vi "new_main_save_encoder.vi"() -> ()   [LabVIEW 2019]
uses:
  <vilib>/vision/Image Controls.llb/IMAQ Image.ctl
  <vilib>/Utility/error.llb/DialogType.ctl
  <vilib>/DAQmx/write.llb/DAQmx Write (Digital Bool 1Line 1Point).vi
  <vilib>/DAQmx/write.llb/DAQmx Write (Counter Frequency 1Chan 1Samp).vi
  <vilib>/Analysis/baseanly.llb/Mean (DBL).vi
  <vilib>/DAQmx/miscellaneous.llb/DAQmx Fill In Error Info.vi
  <vilib>/Utility/file.llb/Write Delimited Spreadsheet (DBL).vi
  <vilib>/addons/control/pid/pid.llb/PID (DBL).vi
  <vilib>/addons/control/pid/pid.llb/PID Gain Schedule (DBL).vi
  <vilib>/DAQmx/create/channels.llb/DAQmx Create Channel (CO-Pulse Generation-Frequency).vi
  <vilib>/DAQmx/configure/timing.llb/DAQmx Timing (Implicit).vi
  <vilib>/vision/driver/NI_Vision_Acquisition_Software.lvlib
  <vilib>/userDefined/High Color/IMAQdx.ctl
  <instrlib>/Yokogawa PZ4000/Yokogawa PZ4000.lvlib
  <vilib>/Analysis/NI_AALBase.lvlib
  <vilib>/addons/control/pid/NI_PID_pid.lvlib
  <instrlib>/Agilent 34970/Agilent 34970.lvlib
  <instrlib>/Yokogawa WT200 Series/Yokogawa WT200 Series.lvlib
  <resource>/objmgr/daqmx.rc
panel:
  in  "encoder files":u32=10
  in  "Salvar encoder":bool
  in  "encoder wait":u32=200
  out "T end ensaio":dbl format="%_19f"
  out "T init ensaio":dbl format="%_19f"
  out "save name":string
  out "Error Out":T1
  out "Torque à vazio":dbl format="%_19f"
  out "error out 3":errorcluster
  out "temperature array cluster":T2
  out "temperature num cluster":T3
  out "watt num cluster":T4
  out "var controle rpm":u16
  out "var controle torque":dbl format="%.2f"
  out "error out 2":errorcluster
  out "watt array cluster":T5
  out "rpm array cluster":T6
  out "rpm values cluster":T7
  out "stop aquisition?":bool
  out "torque values cluster":T8
  out "torque array cluster":T9
  out "lim sup rpm":dbl=250000.0 format="%#_13g"
  out "lim inf rpm":dbl=250000.0 format="%#_13g"
  out "lim inf torque":dbl=250000.0 format="%#_13g"
  out "lim sup torque":dbl=250000.0 format="%#_13g"
  out "t0 ensaio":dbl format="%_19f"
  out "error out":errorcluster
  out "Referência entrada (RPM)":dbl
  out "RPM":dbl
  out "Image Out":T10
  out "torque mean":dbl format="%0.2f"
  out "semaforo medição":T11
  out "Status de execução":string
  out "eixo girando?":bool
  out "Referência entrada (mN.m)":dbl
  out "ME":enum16{"Stand-by", "Ensaiando", "Saindo"}(ring)
  in  "stop geral":bool
  in  "Tab Control":T12(tab)
  in  "manter na condição após ensaio?":bool
  in  "T aquisição":dbl=10.0 format="%#_13g"
  in  "name or relative path":string
  out "Power XY":cluster{dbl[], dbl[]}(graph)
  out "Torque XY":cluster{"t":dbl[], dbl[]}[](graph)
  in  "Torque (mN.m)":dbl min=0.0 max=500.0 step=0.1
  in  "Velocidade angular (RPM)":dbl=1000.0 min=1000.0 max=3600.0 step=0.1
  out "Descrição":string
  in  "Lista de ensaios":T13(ring)
  in  "Iniciar ensaio":bool
  in  "stop ensaio":bool
  in  "Ensaiando?":bool
  out "RPM XY":cluster{"t":dbl[], dbl[]}[](graph)
  in  "Salvar dados":bool
  in  "Tab Control 5":enum32{"RPM", "Torque", "Temperatura"}(tab)
  out "encoder saved":i32
  out "Waveform RPM":dynamicdata(graph)
  out "Waveform Torque":dynamicdata(graph)
  out "Chart Temperatura":cluster{dbl, dbl, dbl, dbl, dbl, dbl}(graph)
  in  "Tab Control 4":enum32{"Numeric - WT230", "Waveform - PZ4000"}(tab)
  out "Chart potencia numeric":T14(graph)
  out "Chart corrente numeric":cluster{"I(A)":dbl, "I(B)":dbl, "I(E)":dbl}(graph)
  out "Chart tensão numeric":cluster{"V(A)":dbl, "V(B)":dbl, "V(E)":dbl}(graph)
  out "Chart Potencia":cluster{dbl, dbl, dbl, dbl}(graph)
  out "Corrente":dbl[][](graph)
  out "Tensão":dbl[][](graph)
  in  "Tab Control 3":T15(tab)
  in  "Tab Control 6":T16(tab)
  in  "Parar motor":bool
  in  "Enviar velocidade":bool
  in  "Velocidade (RPM)":u16=1000 min=1000 max=10000 step=100
  in  "Frequência PWM":u16(ring) items=["2000 Hz", "3600 Hz", "5000 Hz", "8000 Hz"]
  in  "Enviar frequência":bool
  in  "Modo PWM":u16(ring) items=["Standard", "Complete", "Symmetric", "Anti Symmetric"]
  in  "Enviar modo":bool
  out "Tradução":string
  in  "Envia mensagem":bool
  in  "Mensagem":T17(ring)=enum."Read power"
  out "Resposta":string
  in  "Seta carga":bool
  in  "Liga saída":bool
  out "Corrente de saída":dbl format="%.4f"
  out "Tensão de saída":dbl format="%.4f"
  in  "Limite de tensão":dbl=15.0 min=0.0 max=17.0 step=0.5 format="%.4f"
  in  "Limite de corrente":dbl=0.3000000000000001 min=0.0 max=0.4 step=0.01 format="%.4f"
  in  "Tempo de aquisição":u16(ring)=12 items=["1ksec", "400sec", "200sec", "100sec", "40sec", "20sec", "10sec", "4sec", "2sec", "1sec", "400msec", "200msec", "100msec", "40msec", "20msec", "10msec", "4msec", "2msec", "1msec", "400usec", "200usec", "100usec", "40usec", "20usec", "10usec"]
  in  "Waveform?":bool
  in  "Filtro de linha":u16(ring) items=["OFF", "500Hz", "20kHz", "1MHz"]
  in  "Média":u16(ring)=6 items=["2", "4", "8", "16", "32", "64", "OFF"]
  in  "dt integracao":dbl=1.0 format="%#_13g"
  in  "Realiza medição PZ4000":bool
  in  "Medição contínua? PZ4000":bool
  in  "Realiza medição WT230":bool
  in  "Medição contínua? WT230":bool
  in  "Tempo de integração (s)":u32=10 min=1 max=60 step=1
  in  "Liga aquecedor":bool
  in  "Frequency":dbl=1.0 format="%.6f"
  in  "Duty Cycle":dbl=0.225 format="%.6f"
  out "Chart RPM":T18(graph)
  in  "stop manual":bool
  out "Chart Torque":T19(graph)
  in  "Tab Control 2":enum32{"Torque", "Velocidade", "Torque GS"}(tab)
  in  "Habilitar (Torque)":bool
  in  "Referência (mN.m)":dbl min=0.0 max=500.0 step=0.1
  in  "Setar referência (Torque)":bool
  in  "PID Torque":T20={"proportional gain (Kc)"=0.0002, "integral time (Ti, min)"=0.005, "derivative time (Td, min)"=0.0}
  out "torque em rp?":bool
  in  "PID RPM":T20={"proportional gain (Kc)"=0.05, "integral time (Ti, min)"=0.005, "derivative time (Td, min)"=0.0}
  in  "Referência (RPM)":dbl=1000.0 min=900.0 max=5000.0 step=0.1
  in  "Habilitar (RPM)":bool
  in  "Setar referência (RPM)":bool
  out "rpm em rp?":bool
  in  "PID gain schedule":T21(array[cluster])=[{"PID gains"={"proportional gain (Kc)"=0.000167, "integral time (Ti, min)"=0.0048, "derivative time (Td, min)"=0.0}, "max value"=75.0}] {"max value" format="%.2f"; "PID gains"."derivative time (Td, min)" format="%.7f"; "PID gains"."integral time (Ti, min)" format="%.7f"; "PID gains"."proportional gain (Kc)" format="%.7f"}
  in  "waveform file name":string="data_%d%m@%H%M%S.txt"
  in  "Salvar waveform":bool
  in  "Limpa gráficos":bool
  in  "Janela de dados (s)":dbl=600.0
  in  "Iluminação":bool
  out "Image":T10(plugin-control)
  in  "Margem RPM (%)":dbl=0.5 min=0.0 max=2.1 step=0.1
  in  "Margem torque (%)":dbl=0.4999999999999998 min=0.0 max=2.1 step=0.1
  in  "Parâmetros serial":T22={"Serial VCC"="COM5", "timeout"=2, "baud rate"=600, "flow control"=0, "data bits"=8, "parity"=enum."None", "stop bits"=10, "termination char"=FALSE} {"stop bits" items=["1.0"=10, "1.5"=15, "2.0"=20]; "flow control" items=["None", "XON/XOFF", "RTS/CTS", "XON/XOFF & RTS/CTS", "DTR/DSR", "XON/XOFF & DTR/DSR"]}
  in  "RPM Samples (n)":i32=25000
  in  "RPM Rate (Hz)":dbl=500000.0 format="%#_13g"
  in  "Torque Samples (n)":i32=25000
  in  "Torque Rate (Hz)":dbl=500000.0 format="%#_13g"
  in  "Array frequências":u16[](array[ring])=[0, 1, 2, 3] items=["2000 Hz", "3600 Hz", "5000 Hz", "8000 Hz"]
  in  "Array modos":u16[](array[ring])=[0, 2, 3] items=["Standard", "Complete", "Symmetric", "Anti Symmetric"]
  in  "format":string="%.10f"
  # "Parâmetros"
  # "Execução"
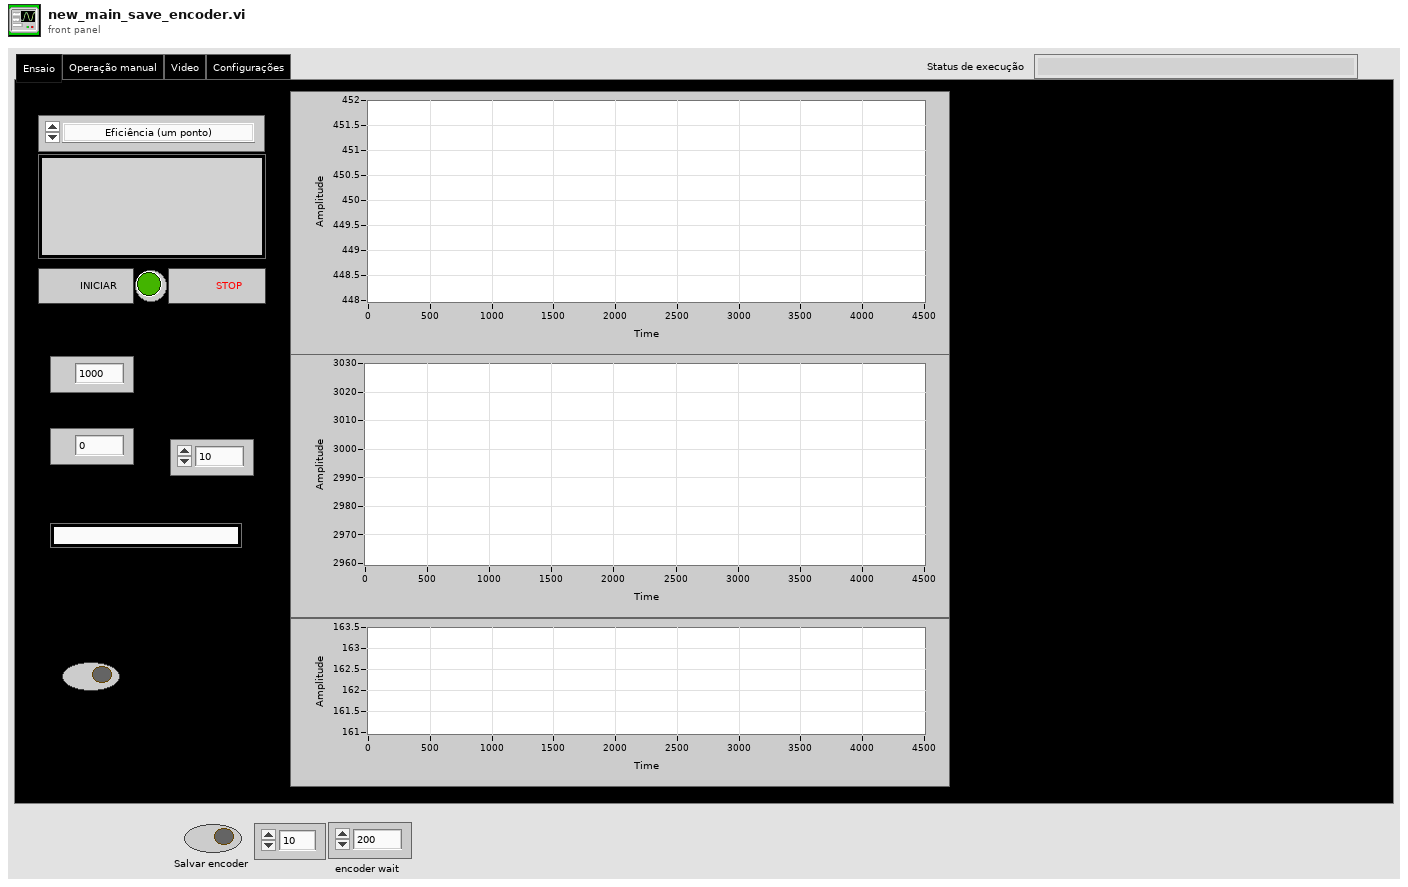
[diagram p1: front panel]
types:
  T1 = cluster{"status":bool, "code":i32, "message":string}
  T2 = cluster{"t":dbl[], "t1 bobina":dbl[], "t2 bobina":dbl[], "t freio":dbl[], "t rola frente":dbl[], "t rola tras":dbl[], "t amb":dbl[], "duty cycle":dbl[]}
  T3 = cluster{"t1 bobina":dbl, "t2 bobina":dbl, "t freio":dbl, "tempo":dbl, "t rola frente":dbl, "t rola tras":dbl, "t amb":dbl, "duty cycle":dbl}
  T4 = cluster{"V(A)":dbl, "I(A)":dbl, "V(B)":dbl, "I(B)":dbl, "PC(A)":dbl, "PC(B)":dbl, "PC(T)":dbl, "PL(T)":dbl, "PL(B)":dbl, "PL(A)":dbl, "V(E)":dbl, "PL(E)":dbl, "PC(E)":dbl, "I(E)":dbl, "t":dbl}
  T5 = cluster{"t":dbl[], "V(A)":dbl[], "I(A)":dbl[], "V(B)":dbl[], "I(B)":dbl[], "PC(A)":dbl[], "PC(B)":dbl[], "PC(T)":dbl[], "PL(T)":dbl[], "PL(B)":dbl[], "PL(A)":dbl[], "V(E)":dbl[], "PL(E)":dbl[], "PC(E)":dbl[], "I(E)":dbl[]}
  T6 = cluster{"t":dbl[], "rpm":dbl[], "ref":dbl[], "lim sup":dbl[], "lim inf":dbl[], "var contr":dbl[]}
  T7 = cluster{"relative seconds":dbl, "RPM":dbl, "Referência entrada (RPM)":dbl, "lim sup rpm":dbl, "lim inf rpm":dbl, "var controle rpm":dbl}
  T8 = cluster{"relative seconds":dbl, "mean":dbl, "Referência entrada (mN.m)":dbl, "lim sup torque":dbl, "lim inf torque":dbl, "var controle torque":dbl}
  T9 = cluster{"t":dbl[], "torque":dbl[], "ref":dbl[], "lim sup":dbl[], "lim inf":dbl[], "var contr":dbl[]}
  T10 = typedef "IMAQ Image.ctl" = refnum<image>
  T11 = typedef "Semaphore RefNum" = refnum<k1>
  T12 = enum32{"Ensaio", "Operação manual", "Video", "Configurações"}
  T13 = enum16{"Eficiência (um ponto)", "Eficiência (um ponto) v2", "Eficiência (múltiplos pontos)"}
  T14 = cluster{"PC(A)":dbl, "PC(B)":dbl, "PC(T)":dbl, "PL(A)":dbl, "PL(B)":dbl, "PL(T)":dbl, "PC(E)":dbl, "PL(E)":dbl}
  T15 = enum32{"Inversor", "Freio", "PZ4000", "WT230", "Aquecimento"}
  T16 = enum32{"Velocidade", "Frequência PWM", "Modo PWM"}
  T17 = enum16{"Read set speed", "Read operation status", "Read power", "Read starting trials", "Read bus voltage", "Read temperature", "Read power limitation", "Read PWM mode", "Read PWM frequency", "Read real speed"}
  T18 = cluster{"RPM":dbl, "Referência entrada (RPM)":dbl, "lim sup rpm":dbl, "lim inf rpm":dbl}
  T19 = cluster{"mean":dbl, "Referência entrada (mN.m)":dbl, "lim sup torque":dbl, "lim inf torque":dbl}
  T20 = cluster{"proportional gain (Kc)":dbl, "integral time (Ti, min)":dbl, "derivative time (Td, min)":dbl}
  T21 = cluster{"PID gains":cluster{"proportional gain (Kc)":dbl, "integral time (Ti, min)":dbl, "derivative time (Td, min)":dbl}, "max value":dbl}[]
  T22 = cluster{"Serial VCC":refnum<visa-resource-name>, "timeout":u32, "baud rate":u32, "flow control":u16, "data bits":u16, "parity":enum16{"None", "Odd", "Even", "Mark", "Space"}, "stop bits":u16, "termination char":bool}
  T23 = enum8{"Enabled", "Disabled", "Disabled and Grayed Out"}
  T24 = enum32{"Page Enabled", "Page Disabled", "Page Disabled & Grayed"}
  T25 = typedef "IMAQdx.ctl" = refnum<k21>
  T26 = enum16{"Start Comm.", "End Comm.", "Wait", "Send Static Message", "Set Speed"}
  T27 = enum16{"Thermocouple", "Thermistor", "RTD", "4-Wire RTD", "Default (Last)"}
  T28 = enum16{"Start Comm.", "End Comm.", "Wait", "Send Static Message", "Set Speed", "Set PWM Mode", "Set PWM Frequency"}
  T29 = enum16{"Read set speed", "Read operation status", "Read power", "Read starting trials", "Read bus voltage", "Read temperature", "Read power limitation", "Read PWM mode", "Read PWM frequency"}
  T30 = cluster{"mean":dbl, "Referência entrada (mN.m)":dbl, "lim sup torque":dbl, "lim inf torque":dbl}[]
  T31 = cluster{"relative seconds":dbl, dbl, "Referência entrada (mN.m)":dbl, "lim sup torque":dbl, "lim inf torque":dbl, "var controle torque":dbl}
  T32 = cluster{dbl, "Referência entrada (mN.m)":dbl, "lim sup torque":dbl, "lim inf torque":dbl}
  T33 = typedef "DialogType.ctl" = u16
  T34 = cluster{"relative seconds":dbl, "RPM":dbl, "Referência entrada (RPM)":dbl, "lim sup rpm":dbl, "lim inf rpm":dbl, "var controle rpm":u16}
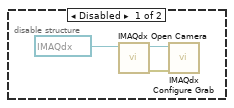
[diagram p3: hidden frame]
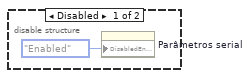
[diagram p4: hidden frame]
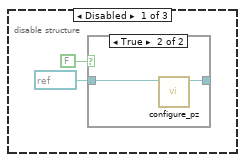
[diagram p5: hidden frame]
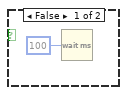
[diagram p8: hidden frame]
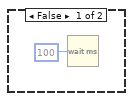
[diagram p9: hidden frame]
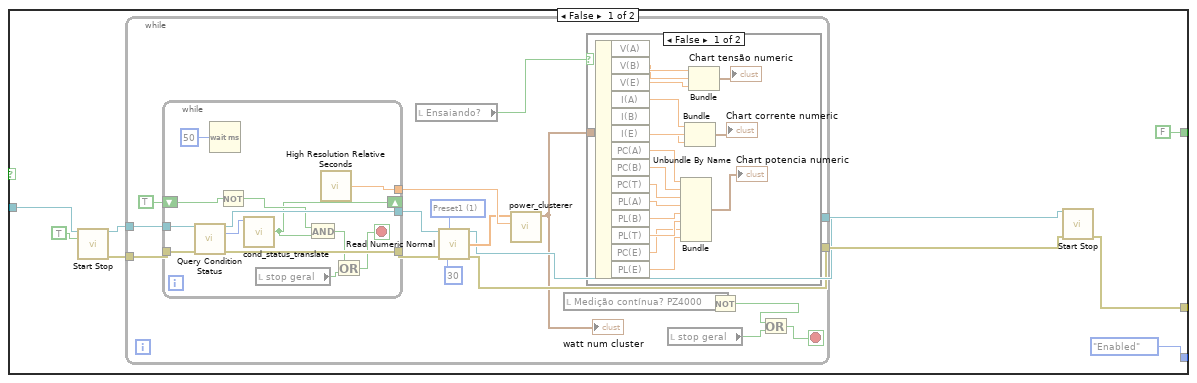
[diagram p10: hidden frame]
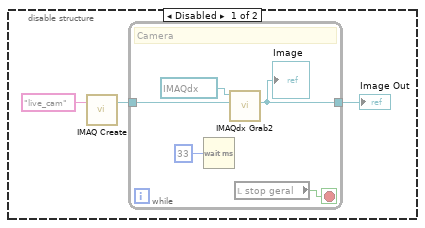
[diagram p13: hidden frame]
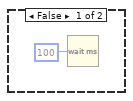
[diagram p14: hidden frame]
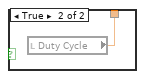
[diagram p16: hidden frame]
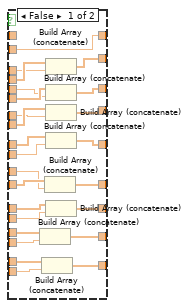
[diagram p18: hidden frame]
diagram:
  n1 = flat-sequence {
    frame #0 {
      "Status de execução" <- "Configurando" ("Status de execução")
      "ME" <- enum16{"Stand-by", "Ensaiando", "Saindo"}."Stand-by" ("ME")
      "Referência entrada (mN.m)" <- 0.0 ("Referência entrada")
      "Referência entrada (RPM)" <- 0.0 ("Referência entrada")
      "Torque à vazio" <- 0.0 ("Torque à vazio")
    }
    frame #1 {
      w11 = T8 {"relative seconds"=nan, "mean"=nan, "Referência entrada (mN.m)"=nan, "lim sup torque"=nan, "lim inf torque"=nan, "var controle torque"=nan} ("torque values cluster")
      w16 = T30 [] ("History Data")
      w21 = T23."Enabled" ("Disabled")
      w22 = 0.0 ("Referência")
      w27 = refnum<k21> "resfriamento_freio"  # DAQmx Task Name
      w6 = FALSE ("data")
      n2 = disable-structure shown="Disabled" {
        frame Disabled {
          n3 = case shown="True" FALSE ("configure?") {
            tunnel: [w52 w54] -> _
            tunnel: refnum<visa-resource-name> "PZ" ("VISA Refnum in") -> [w52 w53]
            frame False {
            }
            frame True {
              n4 = call "configure_pz.vi"("VISA Refnum in"=w53) -> ("VISA Refnum out"=w54:refnum<visa-resource-name>)  [unwired: 10 in]
            }
          }
        }
        frame Enabled {
        }
        frame Disabled {
          w58 = u16 9 items=["AUTO", "0.1", "0.2", "0.4", "1", "2", "4", "10", "20", "40", "100"] ("A Range (7:10)")
          w59 = u16 1 items=["5A", "20A", "Sensor"] ("A Terminal (0: 5A)")
          w60 = u16 6 items=["AUTO", "30", "60", "120", "200", "300", "600", "1200", "2000"] ("V Range (8: 2000)")
          n5 = call <instrlib>:"Initialize.vi"("VISA resource name"=refnum<visa-resource-name> "PZ" ("VISA Refnum in"), "Reset (T: Reset)"=FALSE) -> ("VISA resource name out"=w56:refnum<visa-resource-name>)  [unwired: 12 in, 1 out]
          n6 = call <instrlib>:"Config Voltage.vi"("VISA resource name"=w56, "V Range (8: 2000)"=w60) -> ("VISA resource name out"=w61:refnum<visa-resource-name>)  [unwired: 12 in, 1 out]
          n7 = call <instrlib>:"Config Current.vi"("VISA resource name"=w61, "A Terminal (0: 5A)"=w59, "A Range (7:10)"=w58) -> ()  [unwired: 11 in, 2 out]
        }
      }
      n8 = disable-structure shown="Disabled" {
        frame Disabled {
          w35 = refnum<k21> "iluminacao"  # DAQmx Task Name
          n9 = call <vilib>:"DAQmx Start Task.vi"("task/channels in"=w35) -> ("task out"=w36:refnum<k21>)  [unwired: 13 in, 1 out]
          n10 = call-poly <vilib>:"DAQmx Write.vi"("task/channels in"=w36, "data"=FALSE) -> ()  [unwired: 11 in, 3 out]
        }
        frame Enabled {
        }
      }
      n11 = local write "Referência (mN.m)"(w22) -> ()
      n12 = property on="Tab Control" class="TabCtl (strict)"() -> ("Pages"=w31:refnum<vi>[])  [unwired: 2 in, 2 out]
      n13 = local write "Referência (RPM)"(w22) -> ()
      n14 = Index Array(array=w31, index=1) -> (element=w32:refnum<vi>)
      n15 = property on="Chart Torque" class="WFChart (strict)"("History Data"=w16) -> ()  [unwired: 2 in, 2 out]
      n16 = property class="Page"(reference=w32, "PageEnb"=T24."Page Enabled" ("Page Enabled State")) -> ()  [unwired: 1 in, 2 out]
      n17 = property on="Chart RPM" class="WFChart (strict)"("History Data"=w16) -> ()  [unwired: 2 in, 2 out]
      n18 = local write "torque values cluster"(w11) -> ()
      n19 = local write "rpm values cluster"(w11) -> ()
      n20 = local write "watt num cluster"(T4 {"V(A)"=0.0, "I(A)"=0.0, "V(B)"=0.0, "I(B)"=0.0, "PC(A)"=0.0, "PC(B)"=0.0, "PC(T)"=0.0, "PL(T)"=0.0, "PL(B)"=0.0, "PL(A)"=0.0, "V(E)"=0.0, "PL(E)"=0.0, "PC(E)"=0.0, "I(E)"=0.0, "t"=0.0} ("watt num cluster")) -> ()
      n21 = disable-structure shown="Enabled" {
        frame Disabled {
          n22 = call <vilib>:"IMAQdx Open Camera.vi"("Session In"=T25 "cam0") -> ("error out"=w37:errorcluster, "Session Out"=w38:T25)  [unwired: 9 in]
          n23 = call <vilib>:"IMAQdx Configure Grab.vi"("error in"=w37, "Session In"=w38) -> ()  [unwired: 8 in, 2 out]
        }
        frame Enabled {
        }
      }
      n24 = flat-sequence {
        frame #0 {
          w41 = refnum<k21> "alimentacao_inversor"  # DAQmx Task Name
          n25 = call <vilib>:"DAQmx Start Task.vi"("task/channels in"=w41) -> ("task out"=w43:refnum<k21>)  [unwired: 13 in, 1 out]
          n26 = call-poly <vilib>:"DAQmx Write.vi"("task/channels in"=w43, "data"=TRUE) -> ()  [unwired: 11 in, 3 out]
        }
        frame #1 {
          n27 = Wait (ms)(milliseconds to wait=u32 3000) -> ()  [unwired: 1 out]
        }
        frame #2 {
          n28 = call "Serial_control.vi"("Função"=T26."Start Comm.", "comm cluster"="Parâmetros serial") -> ()  [unwired: 3 in, 4 out]
        }
        frame #3 {
          n29 = local read "Parâmetros serial"() -> (w48:T22)
          n30 = call "Serial_control.vi"("Enviar número"=u16 0, "Função"=T26."Set Speed", "comm cluster"=w48) -> ()  [unwired: 2 in, 4 out]
        }
      }
      n31 = call <vilib>:"Obtain Semaphore Reference.vi"() -> ("semaphore"=→"semaforo medição":T11)  [unwired: 5 in, 2 out]
      n32 = property on="Chart Potencia" class="WFChart (strict)"("History Data"=cluster{dbl, dbl, dbl, dbl}[] []) -> ()  [unwired: 2 in, 2 out]
      n33 = property on="Iniciar ensaio" class="Bool (strict)"("DisabledEnum"=T23."Enabled" ("Disabled")) -> ()  [unwired: 2 in, 2 out]
      n34 = disable-structure shown="Enabled" {
        frame Disabled {
          n35 = property on="Parâmetros serial" class="Clust (strict)"("DisabledEnum"=T23."Enabled" ("Disabled")) -> ()  [unwired: 2 in, 2 out]
        }
        frame Enabled {
        }
      }
      n36 = call <instrlib>:"GENie Initialize.vi"("Reset (T)"=TRUE, "VISA name"=refnum<visa-resource-name> "Lambda") -> ("error out"=w15:errorcluster, "VISA out"=w14:refnum<visa-resource-name>)  [unwired: 8 in]
      n37 = call <instrlib>:"Initialize.vi"("VISA Resource Name"=refnum<visa-resource-name> "Agilent" ("VISA AGILENT"), "Reset (T: Reset)"=TRUE) -> ()  [unwired: 12 in, 2 out]
      n38 = property on="Parâmetros serial" class="Clust (strict)"("DisabledEnum"=T23."Enabled" ("Disabled")) -> ()  [unwired: 2 in, 2 out]
      n39 = call <vilib>:"DAQmx Start Task.vi"("task/channels in"=w27) -> ("task out"=w26:refnum<k21>)  [unwired: 13 in, 1 out]
      n40 = call <instrlib>:"GENie Config Power-On State.vi"("error"=w15, "Power-On"=enum16{"Safe-Start", "Auto-Start"}."Safe-Start", "VISA"=w14) -> ()  [unwired: 7 in, 2 out]
      n41 = call-poly <vilib>:"DAQmx Write.vi"("task/channels in"=w26, "data"=FALSE) -> ()  [unwired: 11 in, 3 out]
      n42 = local write "Realiza medição PZ4000"(w6) -> ()
      n43 = local write "Realiza medição WT230"(w6) -> ()
      n44 = local write "Enviar velocidade"(w6) -> ()
      n45 = local write "stop manual"(w6) -> ()
      n46 = local write "stop ensaio"(w6) -> ()
      n47 = local write "Envia mensagem"(w6) -> ()
      n48 = local write "stop geral"(w6) -> ()
      n49 = local write "Habilitar (RPM)"(w6) -> ()
      n50 = local write "Iluminação"(w6) -> ()
      n51 = local write "Habilitar (Torque)"(w6) -> ()
      n52 = local write "Setar referência (RPM)"(w6) -> ()
      n53 = local write "eixo girando?"(w6) -> ()
      n54 = local write "Waveform?"(w6) -> ()
      n55 = local write "Setar referência (Torque)"(w6) -> ()
      n56 = local write "rpm em rp?"(w6) -> ()
      n57 = local write "torque em rp?"(w6) -> ()
      n58 = local write "Parar motor"(w6) -> ()
      n59 = local write "Limpa gráficos"(w6) -> ()
      n60 = local write "Liga saída"(w6) -> ()
      n61 = local write "Ensaiando?"(w6) -> ()
      n62 = local write "Seta carga"(w6) -> ()
      n63 = local write "Liga aquecedor"(w6) -> ()
      n64 = local write "stop aquisition?"(w6) -> ()
      n65 = local write "Medição contínua? PZ4000"(w6) -> ()
      n66 = local write "Salvar waveform"(w6) -> ()
      n67 = property on="Liga saída" class="Bool (strict)"("DisabledEnum"=w21) -> ()  [unwired: 2 in, 2 out]
      n68 = property on="Parar motor" class="Bool (strict)"("DisabledEnum"=w21) -> ()  [unwired: 2 in, 2 out]
      n69 = property on="Velocidade (RPM)" class="DigNum (strict)"("DisabledEnum"=w21) -> ()  [unwired: 2 in, 2 out]
      n70 = property on="Enviar velocidade" class="Bool (strict)"("DisabledEnum"=w21) -> ()  [unwired: 2 in, 2 out]
      n71 = property on="Seta carga" class="Bool (strict)"("DisabledEnum"=w21) -> ()  [unwired: 2 in, 2 out]
      n72 = property on="Tempo de aquisição" class="Ring (strict)"("Maximum"=18.0 ("Data Entry Limits:Maximum"), "Minimum"=0.0 ("Data Entry Limits:Minimum"), "Disabled Items []"=i32[] [19, 20, 21, 22, 23, 24]) -> ()  [unwired: 2 in, 2 out]
      n73 = property on="Realiza medição WT230" class="Bool (strict)"("DisabledEnum"=T23."Enabled" ("Disabled")) -> ()  [unwired: 2 in, 2 out]
    }
    frame #2 {
      w63 = dbl[] []
      w66 = dbl[] []
      w68 = dbl[] []
      w71 = dbl[] []
      n74 = disable-structure shown="Enabled" {
        frame Disabled {
          n75 = call "IMAQ Create"("Image Name"="live_cam") -> ("New Image"=w228:T10)  [unwired: 3 in, 2 out]
          n76 = while {
            tunnel: w228 -> [w232]
            tunnel: [w230] -> w227
            stop <- w231 stop-if-true
            # "Camera"
            n77 = Wait (ms)(milliseconds to wait=u32 33) -> ()  [unwired: 1 out]
            n78 = call <vilib>:"IMAQdx Grab2.vi"("Image In"=w232, "Session In"=T25 "cam0") -> ("Image Out"=w230:T10)  [unwired: 6 in, 3 out]
            "Image" <- w230
            n79 = local read "stop geral"() -> (w231:bool)
          }
          "Image Out" <- w227
        }
        frame Enabled {
        }
      }
      n80 = while {
        stop <- w850 stop-if-true
        # "Aquisição - Torque"
        n81 = flat-sequence {
          tunnel: [w863] -> w851
          tunnel: [w868] -> w853
          tunnel: [w867] -> w852
          tunnel: w851 -> [w867]
          tunnel: [w864] -> w846
          tunnel: w853 -> [w869]
          tunnel: w852 -> [w870]
          tunnel: [w869] -> w837
          frame #0 {
            n82 = local read "semaforo medição"() -> (w862:T11)
            n83 = call <vilib>:"Acquire Semaphore.vi"("semaphore"=w862) -> ("semaphore out"=w863:T11)  [unwired: 4 in, 2 out]
          }
          frame #1 {
            n84 = call "DAQ Assistant"("rate"="Torque Rate (Hz)", "number of samples"="Torque Samples (n)") -> ("data"=w868:dynamicdata)  [unwired: 15 in, 2 out]
            n85 = call <vilib>:"High Resolution Relative Seconds.vi"() -> ("relative seconds"=w864:dbl)
          }
          frame #2 {
            n86 = call <vilib>:"Release Semaphore.vi"("semaphore"=w870) -> ()  [unwired: 5 in, 2 out]
          }
        }
        n87 = local read "Habilitar (Torque)"() -> (w849:bool)
        n88 = case shown="False" w849 {
          tunnel: [w857 w861] -> w845
          tunnel: [w857 w860] -> w844
          tunnel: [w857 w859] -> w843
          tunnel: [w856 w858] -> w841
          frame False {
            w857 = nan
            n89 = local read "Corrente de saída"() -> (w856:dbl)
          }
          frame True {
            n90 = local read "Referência entrada (mN.m)"() -> (w861:dbl)
            n91 = local read "var controle torque"() -> (w858:dbl)
            n92 = local read "lim sup torque"() -> (w860:dbl)
            n93 = local read "lim inf torque"() -> (w859:dbl)
          }
        }
        n94 = local read "Torque à vazio"() -> (w838:dbl)
        n95 = call "Convert from Dynamic Data"("Dynamic Data Type"=w837) -> ("Array"=w854:dbl[])  [unwired: 3 in]
        n96 = call-poly <vilib>:"Mean.vi"("X"=w854) -> ("mean"=w839:dbl)  [unwired: 1 out]
        n97 = Subtract(x=w839, y=w838) -> (x-y=w840:dbl)
        "torque mean" <- w840
        n98 = local read "Ensaiando?"() -> (w848:bool)
        n99 = Bundle("relative seconds"=w846, w840, "Referência entrada (mN.m)"=w845, "lim sup torque"=w844, "lim inf torque"=w843, "var controle torque"=w841) -> (→"torque values cluster":T31)  [unwired: 1 in]
        n100 = Bundle(w840, "Referência entrada (mN.m)"=w845, "lim sup torque"=w844, "lim inf torque"=w843) -> (w847:T32)  [unwired: 1 in]
        n101 = case shown="False" w848 {
          tunnel: w847 -> [w855 _]
          frame False {
            "Chart Torque" <- w855
          }
          frame True {
          }
        }
        n102 = local read "stop geral"() -> (w850:bool)
        "Waveform Torque" <- w837
      }
      n103 = while {
        tunnel: refnum<visa-resource-name> "Agilent" ("VISA Resource Name") -> [w305]
        stop <- w301 stop-if-true
        # "Aquisição - Temperatura"
        n104 = local read "stop geral"() -> (w301:bool)
        n105 = local read "Liga aquecedor"() -> (w286:bool)
        n106 = Wait (ms)(milliseconds to wait=u32 5000 ("millisecond multiple")) -> ()  [unwired: 1 out]
        n107 = call <instrlib>:"EZ Temperature.vi"("VISA Resource Name"=w305, "Scan List (empty)"="101,102,103, 104, 105, 106", "Transducer Type (4:Def-Last)"=T27."4-Wire RTD") -> ("Output Array"=w304:dbl[], "error out"=→"error out 3":errorcluster)  [unwired: 10 in, 1 out]
        n108 = case shown="False" w286 {
          tunnel: [0.0 ("Duty Cycle") w310] -> w284
          frame False {
          }
          frame True {
            n109 = local read "Duty Cycle"() -> (w310:dbl)
          }
        }
        n110 = Index Array(array=w304, index #1=0 ("index"), index #2=1 ("index"), index #3=2 ("index"), index #4=3 ("index"), index #5=4 ("index"), index #6=5 ("index")) -> (element #1=w299:dbl, element #2=w297:dbl, element #3=w298:dbl, element #4=w290:dbl, element #5=w289:dbl, element #6=w283:dbl)
        n111 = call <vilib>:"High Resolution Relative Seconds.vi"() -> ("relative seconds"=w291:dbl)
        n112 = local read "Ensaiando?"() -> (w300:bool)
        n113 = Bundle(cluster=T3 {"t1 bobina"=0.0, "t2 bobina"=0.0, "t freio"=0.0, "tempo"=0.0, "t rola frente"=0.0, "t rola tras"=0.0, "t amb"=0.0, "duty cycle"=0.0} ("temperature num cluster 2"), "t1 bobina"=w299, "t2 bobina"=w297, "t freio"=w298, "tempo"=w291, "t rola frente"=w290, "t rola tras"=w289, "t amb"=w283, "duty cycle"=w284) -> (→"temperature num cluster":T3)
        n114 = Bundle(w299, w297, w298, w290, w289, w283) -> (w296:cluster{dbl, dbl, dbl, dbl, dbl, dbl})  [unwired: 1 in]
        n115 = case shown="False" w300 {
          tunnel: w296 -> [w311 _]
          frame False {
            "Chart Temperatura" <- w311
          }
          frame True {
          }
        }
      }
      n116 = while {
        tunnel: refnum<visa-resource-name> "Lambda" ("VISA name") -> [w1257]
        stop <- w1258 stop-if-true
        # "Tratador de eventos"
        n117 = event shown="[7] \"Envia mensagem\": Value Change" {
          selector: _ -> [_ _ _ _ _ _ _ _ _ _ _ _ _ _ _ _ _ _ _ _ _ _]
          dyn-events: _ -> [_ _ _ _ _ _ _ _ _ _ _ _ _ _ _ _ _ _ _ _ _ _]
          timeout: _ -> [_ _ _ _ _ _ _ _ _ _ _ _ _ _ _ _ _ _ _ _ _ _]
          tunnel: w1257 -> [_ _ _ _ _ _ _ _ w1295 w1301 _ _ _ _ _ _ _ _ _ _ _ _]
          tunnel: [w1259 w1260 _ _ _ _ _ _ _ _ _ _ _ _ _ _ _ _ _ _ _ _] -> w1258
          event "stop manual": Value Change {
            n118 = event-data() -> ("NewVal"=w1259:bool)  [unwired: 1 in, 5 out]
            n119 = local write "stop geral"(w1259) -> ()
          }
          event "stop ensaio": Value Change {
            n120 = event-data() -> ("NewVal"=w1260:bool)  [unwired: 1 in, 5 out]
            n121 = local write "stop geral"(w1260) -> ()
          }
          event "Iluminação": Value Change {
            n122 = event-data() -> ("NewVal"=w1261:bool)  [unwired: 1 in, 5 out]
            n123 = disable-structure shown="Disabled" {
              disable-tunnel: w1261 -> [w1262 _]
              frame Disabled {
                w1263 = refnum<k21> "iluminacao"  # DAQmx Task Name
                n124 = call-poly <vilib>:"DAQmx Write.vi"("task/channels in"=w1263, "data"=w1262) -> ()  [unwired: 11 in, 3 out]
              }
              frame Enabled {
              }
            }
          }
          event "Enviar velocidade": Value Change {
            n125 = event-data() -> ("OldVal"=w1269:bool)  [unwired: 1 in, 5 out]
            n126 = local read "Parâmetros serial"() -> (w1268:T22)
            n127 = local write "Enviar velocidade"(w1269) -> ()
            n128 = call "Serial_control.vi"("Enviar número"="Velocidade (RPM)", "Função"=T26."Set Speed", "comm cluster"=w1268) -> ("translated message"=w1265:string, "read buffer"=w1266:string)  [unwired: 2 in, 2 out]
            n129 = local write "Resposta"(w1266) -> ()
            n130 = local write "Tradução"(w1265) -> ()
          }
          event "Enviar frequência": Value Change {
            n131 = event-data() -> ("OldVal"=w1275:bool)  [unwired: 1 in, 5 out]
            n132 = local read "Parâmetros serial"() -> (w1274:T22)
            n133 = local write "Enviar frequência"(w1275) -> ()
            n134 = call "Serial_control.vi"("Enviar número"="Frequência PWM", "Função"=T28."Set PWM Frequency", "comm cluster"=w1274) -> ("translated message"=w1272:string, "read buffer"=w1273:string)  [unwired: 2 in, 2 out]
            n135 = local write "Resposta"(w1273) -> ()
            n136 = local write "Tradução"(w1272) -> ()
          }
          event "Enviar modo": Value Change {
            n137 = event-data() -> ("OldVal"=w1281:bool)  [unwired: 1 in, 5 out]
            n138 = local read "Parâmetros serial"() -> (w1280:T22)
            n139 = local write "Enviar modo"(w1281) -> ()
            n140 = call "Serial_control.vi"("Enviar número"="Modo PWM", "Função"=T28."Set PWM Mode", "comm cluster"=w1280) -> ("translated message"=w1278:string, "read buffer"=w1279:string)  [unwired: 2 in, 2 out]
            n141 = local write "Resposta"(w1279) -> ()
            n142 = local write "Tradução"(w1278) -> ()
          }
          event "Parar motor": Value Change {
            n143 = event-data() -> ("OldVal"=w1284:bool)  [unwired: 1 in, 5 out]
            n144 = local write "Parar motor"(w1284) -> ()
            n145 = local read "Parâmetros serial"() -> (w1287:T22)
            n146 = call "Serial_control.vi"("Enviar número"=u16 0, "Função"=T26."Set Speed", "comm cluster"=w1287) -> ("translated message"=w1282:string, "read buffer"=w1283:string)  [unwired: 2 in, 2 out]
            n147 = local write "Resposta"(w1283) -> ()
            n148 = local write "Tradução"(w1282) -> ()
          }
          event "Envia mensagem": Value Change {
            n149 = event-data() -> ("OldVal"=w1293:bool)  [unwired: 1 in, 5 out]
            n150 = local write "Envia mensagem"(w1293) -> ()
            n151 = local read "Parâmetros serial"() -> (w1292:T22)
            n152 = call "Serial_control.vi"("Message"="Mensagem", "Função"=T26."Send Static Message", "comm cluster"=w1292) -> ("translated message"=w1290:string, "read buffer"=w1289:string)  [unwired: 2 in, 2 out]
            n153 = local write "Resposta"(w1289) -> ()
            n154 = local write "Tradução"(w1290) -> ()
          }
          event "Seta carga": Value Change {
            n155 = event-data() -> ("OldVal"=w1296:bool)  [unwired: 1 in, 6 out]
            n156 = local write "Seta carga"(w1296) -> ()
            n157 = call <instrlib>:"GENie Config Current Limit.vi"("Current Limit"="Limite de corrente", "VISA"=w1295) -> ("VISA out"=w1294:refnum<visa-resource-name>)  [unwired: 8 in, 1 out]
            n158 = call <instrlib>:"GENie Config Voltage Limit.vi"("Volt Limit"="Limite de tensão", "VISA"=w1294) -> ()  [unwired: 8 in, 2 out]
          }
          event "Liga saída": Value Change {
            w1300 = refnum<k21> "resfriamento_freio"  # DAQmx Task Name
            n159 = event-data() -> ("NewVal"=w1299:bool)  [unwired: 1 in, 5 out]
            n160 = call <instrlib>:"GENie Config Output On-Off.vi"("Output ON"=w1299, "VISA"=w1301) -> ()  [unwired: 8 in, 2 out]
            n161 = call-poly <vilib>:"DAQmx Write.vi"("task/channels in"=w1300, "data"=w1299) -> ()  [unwired: 11 in, 3 out]
          }
          event "Setar referência (Torque)": Value Change {
            n162 = event-data() -> ("OldVal"=w1302:bool)  [unwired: 1 in, 5 out]
            n163 = local read "Referência (mN.m)"() -> (w1303:dbl)
            n164 = local write "Setar referência (Torque)"(w1302) -> ()
            n165 = local write "Referência entrada (mN.m)"(w1303) -> ()
          }
          event "Habilitar (Torque)": Value Change {
            n166 = event-data() -> ("NewVal"=w1305:bool)  [unwired: 1 in, 5 out]
            n167 = case shown="True" w1305 {
              tunnel: [T23."Enabled" ("Disabled") T23."Disabled and Grayed Out" ("Disabled")] -> w1304
              frame False {
              }
              frame True {
              }
            }
            n168 = local write "Habilitar (Torque)"(w1305) -> ()
            n169 = property on="Liga saída" class="Bool (strict)"("DisabledEnum"=w1304) -> ()  [unwired: 2 in, 2 out]
            n170 = property on="Seta carga" class="Bool (strict)"("DisabledEnum"=w1304) -> ()  [unwired: 2 in, 2 out]
          }
          event "Setar referência (RPM)": Value Change {
            n171 = event-data() -> ("OldVal"=w1308:bool)  [unwired: 1 in, 5 out]
            n172 = local read "Referência (RPM)"() -> (w1309:dbl)
            n173 = local write "Setar referência (RPM)"(w1308) -> ()
            n174 = local write "Referência entrada (RPM)"(w1309) -> ()
          }
          event "Habilitar (RPM)": Value Change {
            n175 = event-data() -> ("NewVal"=w1311:bool)  [unwired: 1 in, 5 out]
            n176 = case shown="False" w1311 {
              tunnel: [T23."Enabled" ("Disabled") T23."Disabled and Grayed Out" ("Disabled")] -> w1310
              frame False {
              }
              frame True {
              }
            }
            n177 = local write "Habilitar (RPM)"(w1311) -> ()
            n178 = property on="Parar motor" class="Bool (strict)"("DisabledEnum"=w1310) -> ()  [unwired: 2 in, 2 out]
            n179 = property on="Velocidade (RPM)" class="DigNum (strict)"("DisabledEnum"=w1310) -> ()  [unwired: 2 in, 2 out]
            n180 = property on="Enviar velocidade" class="Bool (strict)"("DisabledEnum"=w1310) -> ()  [unwired: 2 in, 2 out]
          }
          event "Limpa gráficos": Value Change {
            w1314 = T30 [] ("History Data")
            n181 = event-data() -> ("OldVal"=w1315:bool)  [unwired: 1 in, 5 out]
            n182 = local write "Limpa gráficos"(w1315) -> ()
            n183 = property on="Chart Torque" class="WFChart (strict)"("History Data"=w1314) -> ()  [unwired: 2 in, 2 out]
            n184 = property on="Chart Potencia" class="WFChart (strict)"("History Data"=w1314) -> ()  [unwired: 2 in, 2 out]
            n185 = property on="Chart RPM" class="WFChart (strict)"("History Data"=w1314) -> ()  [unwired: 2 in, 2 out]
          }
          event "Tempo de aquisição": Value Change {
            n186 = event-data() -> ("NewVal"=w1316:u16)  [unwired: 1 in, 5 out]
            n187 = call <instrlib>:"Config Observation Time.vi"("VISA resource name"=refnum<visa-resource-name> "PZ", "Observation Time (12: 100msec)"=w1316) -> ()  [unwired: 12 in, 2 out]
          }
          event "Filtro de linha": Value Change {
            n188 = event-data() -> ("NewVal"=w1319:u16)  [unwired: 1 in, 5 out]
            n189 = call <instrlib>:"Config Line Filter and Zero Cross.vi"("VISA resource name"=refnum<visa-resource-name> "PZ", "Line Filter (0: OFF)"=w1319) -> ()  [unwired: 12 in, 2 out]
          }
          event "Média": Value Change {
            n190 = event-data() -> ("NewVal"=w1320:u16)  [unwired: 1 in, 5 out]
            n191 = Not Equal?(x=u16 6, y=w1320) -> (x != y?=w1321:bool)
            n192 = case shown="True" w1321 {
              selector: w1321 -> [w1327 w1329]
              tunnel: [w1327 w1329] -> w1324
              tunnel: [u16 0 ("x") w1328] -> w1323
              tunnel: w1320 -> [_ w1328]
              frame False {
              }
              frame True {
              }
            }
            n193 = call <instrlib>:"Config Measure Average.vi"("VISA resource name"=refnum<visa-resource-name> "PZ", "Average (F: OFF)"=w1324, "Average Count (0: 2)"=w1323) -> ()  [unwired: 11 in, 2 out]
          }
          event "Waveform?": Value Change {
            n194 = event-data() -> ("NewVal"=w1330:bool)  [unwired: 1 in, 5 out]
            n195 = local write "Waveform?"(w1330) -> ()
            n196 = case shown="False" w1330 {
              tunnel: [18.0 ("Data Entry Limits:Maximum") 24.0 ("Data Entry Limits:Maximum")] -> w1333
              tunnel: [0.0 ("Data Entry Limits:Minimum") 6.0 ("Data Entry Limits:Minimum")] -> w1332
              tunnel: [i32[] [19, 20, 21, 22, 23, 24] ("Disabled Items []") i32[] [0, 1, 2, 3, 4, 5] ("Disabled Items []")] -> w1331
              frame False {
              }
              frame True {
              }
            }
            n197 = property on="Tempo de aquisição" class="Ring (strict)"("Maximum"=w1333, "Minimum"=w1332, "Disabled Items []"=w1331) -> ()  [unwired: 2 in, 2 out]
          }
          event "Iniciar ensaio": Value Change {
            n198 = event-data() -> ("NewVal"=w1341:bool)  [unwired: 1 in, 5 out]
            n199 = local write "Ensaiando?"(w1341) -> ()
            n200 = property on="Iniciar ensaio" class="Bool (strict)"("DisabledEnum"=T23."Disabled and Grayed Out" ("Disabled")) -> ()  [unwired: 2 in, 2 out]
          }
          event "Salvar dados": Value Change {
            n201 = event-data() -> ("OldVal"=w1364:bool)  [unwired: 1 in, 5 out]
            n202 = call <vilib>:"High Resolution Relative Seconds.vi"() -> ("relative seconds"=w1347:dbl)
            n203 = Subtract(x=w1347, y="Janela de dados (s)") -> (x-y=w1345:dbl)
            n204 = local read "temperature array cluster"() -> (w1342:T2)
            n205 = local write "Salvar dados"(w1364) -> ()
            n206 = local read "torque array cluster"() -> (w1353:T9)
            n207 = local read "rpm array cluster"() -> (w1354:T6)
            n208 = local read "watt array cluster"() -> (w1352:T5)
            n209 = call "rpm_decluster_by_time.vi"("t_init"=w1345, "rpm array cluster"=w1354) -> ("Dados"=w1362:dbl[][], "Tempo"=w1363:dbl[])  [unwired: 8 in]
            n210 = call "torque_decluster_by_time.vi"("t_init"=w1345, "torque array cluster"=w1353) -> ("Dados"=w1360:dbl[][], "Tempo"=w1361:dbl[])  [unwired: 8 in]
            n211 = call "watt_decluster_by_time.vi"("t_init"=w1345, "watt array cluster"=w1352) -> ("Dados"=w1358:dbl[][], "Tempo"=w1359:dbl[])  [unwired: 8 in]
            n212 = call "temperature_decluster_by_time.vi"("t_init"=w1345, "temperature array cluster"=w1342) -> ("Dados"=w1350:dbl[][], "Tempo"=w1351:dbl[])  [unwired: 8 in]
            n213 = Build Array (concatenate)(w1363, w1362, w1361, w1360, w1359, w1358, w1351, w1350) -> (w1357:dbl[][])
            n214 = Format Date/Time String(time format string (%c)="data_%d%m@%H%M%S.txt") -> (date/time string=w1344:string)  [unwired: 2 in]
            n215 = Transpose 2D Array(2D array=w1357) -> (transposed array=w1356:dbl[][])
            n216 = Build Path(base path=path "C:/Users/zomer/Desktop/zomer/LabVIEW/dyna_liae/ensaios/dados avulsos" ("file path (dialog if empty)"), name or relative path=w1344) -> (appended path=w1355:path)
            n217 = call-poly <vilib>:"Write Delimited Spreadsheet.vi"("file path (dialog if empty)"=w1355, "format (%.3f)"="%.6f", "2D data"=w1356) -> ()  [unwired: 11 in, 2 out]
          }
          event "Salvar waveform": Value Change {
            n218 = event-data() -> ("OldVal"=w1376:bool)  [unwired: 1 in, 5 out]
            n219 = local write "Salvar waveform"(w1376) -> ()
            n220 = local read "Tensão"() -> (w1374:dbl[][])
            n221 = call <instrlib>:"Read Sample Rate.vi"("VISA resource name"=refnum<visa-resource-name> "PZ") -> ("Delta T"=w1373:dbl)  [unwired: 12 in, 2 out]
            n222 = local read "Corrente"() -> (w1371:dbl[][])
            n223 = call "create_timevector.vi"("Delta T"=w1373, "Entrada"=w1374) -> ("Ramp Pattern"=w1372:dbl[])  [unwired: 9 in]
            n224 = Build Array (concatenate)(w1372, w1374, w1371) -> (w1370:dbl[][])
            n225 = Transpose 2D Array(2D array=w1370) -> (transposed array=w1369:dbl[][])
            n226 = Build Path(base path=path "C:/Users/zomer/Desktop/zomer/LabVIEW/dyna_liae/ensaios/waveforms" ("file path (dialog if empty)"), name or relative path="waveform file name") -> (appended path=w1368:path)
            n227 = call-poly <vilib>:"Write Delimited Spreadsheet.vi"("file path (dialog if empty)"=w1368, "format (%.3f)"="format", "2D data"=w1369) -> ()  [unwired: 11 in, 2 out]
          }
        }
      }
      n228 = while {
        tunnel: refnum<visa-resource-name> "Lambda" ("VISA name") -> [w872]
        stop <- w871 stop-if-true
        # "Aquisição - Fonte DC"
        n229 = call <instrlib>:"GENie Meas Output Voltage.vi"("VISA"=w872) -> ("Output Voltage"=→"Tensão de saída":dbl, "VISA out"=w875:refnum<visa-resource-name>)  [unwired: 8 in, 1 out]
        n230 = Wait (ms)(milliseconds to wait=u32 100) -> ()  [unwired: 1 out]
        n231 = call <instrlib>:"GENie Meas Output Current.vi"("VISA"=w875) -> ("Output Current"=→"Corrente de saída":dbl)  [unwired: 8 in, 2 out]
        n232 = local read "stop geral"() -> (w871:bool)
      }
      n233 = while {
        stop <- w753 stop-if-true
        # "Aquisição - Wattímetro WT230"
        n234 = local read "Realiza medição WT230"() -> (w754:bool)
        n235 = case shown="True" w754 {
          frame False {
            n236 = Wait (ms)(milliseconds to wait=u32 100) -> ()  [unwired: 1 out]
          }
          frame True {
            n237 = flat-sequence {
              frame #0 {
                n238 = property on="Realiza medição WT230" class="Bool (strict)"("DisabledEnum"=T23."Disabled and Grayed Out" ("Disabled")) -> ()  [unwired: 2 in, 2 out]
              }
              frame #1 {
                w759 = u16 0 items=["Normal", "Continuous"] ("Integ Mode (0: Normal)")
                w760 = u32 0 ("Hour (0)")
                n239 = call <instrlib>:"Config Integration.vi"("VISA resource name"=refnum<visa-resource-name> "WT", "Integ Mode (0: Normal)"=w759, "Hour (0)"=w760, "Minute (0)"=w760, "Second (0)"="Tempo de integração (s)") -> ("VISA resource name out"=w762:refnum<visa-resource-name>, "error out"=w761:errorcluster)  [unwired: 9 in]
                n240 = while {
                  shift-right: [w766] -> _
                  shift-left: w762 -> [w764]
                  shift-right: [w765] -> _
                  shift-left: w761 -> [w763]
                  stop <- w767 stop-if-true
                  w773 = u16 1 items=["Clear", "Normal", "Integrate"] ("Preset Pattern (0: Clear)")
                  n241 = local read "Medição contínua? WT230"() -> (w769:bool)
                  n242 = local read "stop geral"() -> (w770:bool)
                  n243 = call <instrlib>:"Config Measure Preset Normal.vi"("VISA resource name"=w764, "Preset Pattern (0: Clear)"=w773, "error in (no error)"=w763) -> ("VISA resource name out"=w775:refnum<visa-resource-name>, "error out"=w774:errorcluster)  [unwired: 11 in]
                  n244 = Not(x=w769) -> (.not. x?=w768:bool)
                  n245 = Or(x=w768, y=w770) -> (x .or. y?=w767:bool)
                  n246 = call <instrlib>:"Start Stop Integration.vi"("VISA resource name"=w775, "Start/Stop (F: Stop)"=TRUE, "error in (no error)"=w774) -> ("VISA resource name out"=w778:refnum<visa-resource-name>, "error out"=w777:errorcluster)  [unwired: 11 in]
                  n247 = while {
                    shift-left: w778 -> [w813]
                    shift-right: [w801] -> w772
                    shift-left: w777 -> [w810]
                    shift-right: [w799] -> w771
                    stop <- w809 continue-if-true
                    w816 = u16 2  # Integration indicated bit
                    # "mudei de 500 pra 1000"
                    n248 = call <instrlib>:"Read Measure.vi"("VISA resource name"=w813, "error in (no error)"=w810) -> ("VISA resource name out"=w812:refnum<visa-resource-name>, "Measure Value"=w803:sgl[], "error out"=w811:errorcluster)  [unwired: 10 in, 1 out]
                    n249 = call <instrlib>:"Query Condition Status.vi"("VISA resource name"=w812, "error in (no error)"=w811) -> ("VISA resource name out"=w798:refnum<visa-resource-name>, "Condition"=w814:u16, "error out"=w797:errorcluster)  [unwired: 11 in]
                    n250 = And(x=w814, y=w816) -> (x .and. y?=w815:u16)
                    n251 = Not Equal To 0?(x=w815) -> (x != 0?=w809:bool)
                    n252 = case shown="False" w809 {
                      tunnel: [w827 w834] -> w808
                      tunnel: [w826 w834] -> w807
                      tunnel: [w825 w834] -> w806
                      tunnel: [w824 w834] -> w805
                      tunnel: [w823 w833] -> w802
                      tunnel: [w822 w832] -> w800
                      tunnel: w798 -> [w821 w833]
                      tunnel: w797 -> [w820 w832]
                      frame False {
                        w828 = u16 2 items=["Clear", "Normal", "Integrate"] ("Preset Pattern (0: Clear)")
                        n253 = call <instrlib>:"Config Measure Preset Normal.vi"("VISA resource name"=w821, "Preset Pattern (0: Clear)"=w828, "error in (no error)"=w820) -> ("VISA resource name out"=w831:refnum<visa-resource-name>, "error out"=w830:errorcluster)  [unwired: 11 in]
                        n254 = call <instrlib>:"Read Measure.vi"("VISA resource name"=w831, "error in (no error)"=w830) -> ("VISA resource name out"=w823:refnum<visa-resource-name>, "Measure Value"=w829:sgl[], "error out"=w822:errorcluster)  [unwired: 10 in, 1 out]
                        n255 = call "integration_translator.vi"("Valores integração"=w829) -> ("PI(E)"=w824:sgl, "PI(T)"=w825:sgl, "PI(B)"=w826:sgl, "PI(A)"=w827:sgl)  [unwired: 7 in]
                        n256 = Bundle("PI(A)"=w827, "PI(B)"=w826, "PI(T)"=w825, "PI(E)"=w824) -> ()  [unwired: 1 in, 1 out]
                      }
                      frame True {
                        w834 = nan
                      }
                    }
                    n257 = stacked-sequence {
                      tunnel: w802 -> [w818]
                      tunnel: [w818] -> w801
                      tunnel: w800 -> [w817]
                      tunnel: [w817] -> w799
                      frame #0 {
                        w819 = u32 1000  # Interval
                        n258 = Wait (ms)(milliseconds to wait=w819) -> ()  [unwired: 1 out]
                      }
                    }
                    n259 = call <vilib>:"High Resolution Relative Seconds.vi"() -> ("relative seconds"=w804:dbl)
                    n260 = call "measurements_to_cluster.vi"("PI(E)"=w805, "PI(T)"=w806, "relative seconds"=w804, "PI(B)"=w807, "PI(A)"=w808, "Measure Value"=w803) -> ("watt cluster"=w783:T4)  [unwired: 4 in, 1 out]
                    n261 = local write "watt num cluster"(w783) -> ()
                    n262 = Unbundle By Name(w783) -> ("V(A)"=w796:dbl, "V(B)"=w784:dbl, "V(E)"=w785:dbl, "I(A)"=w786:dbl, "I(B)"=w787:dbl, "I(E)"=w788:dbl, "PC(A)"=w789:dbl, "PC(B)"=w790:dbl, "PC(T)"=w791:dbl, "PL(A)"=w792:dbl, "PL(B)"=w793:dbl, "PL(T)"=w794:dbl, "PC(E)"=w795:dbl, "PL(E)"=w782:dbl)
                    n263 = Bundle("PC(A)"=w789, "PC(B)"=w790, "PC(T)"=w791, "PL(A)"=w792, "PL(B)"=w793, "PL(T)"=w794, "PC(E)"=w795, "PL(E)"=w782) -> (w780:T14)  [unwired: 1 in]
                    n264 = Bundle("I(A)"=w786, "I(B)"=w787, "I(E)"=w788) -> (w779:cluster{"I(A)":dbl, "I(B)":dbl, "I(E)":dbl})  [unwired: 1 in]
                    n265 = Bundle("V(A)"=w796, "V(B)"=w784, "V(E)"=w785) -> (w781:cluster{"V(A)":dbl, "V(B)":dbl, "V(E)":dbl})  [unwired: 1 in]
                    n266 = local write "Chart potencia numeric"(w780) -> ()
                    n267 = local write "Chart tensão numeric"(w781) -> ()
                    n268 = local write "Chart corrente numeric"(w779) -> ()
                  }
                  n269 = call <instrlib>:"Reset Integration.vi"("VISA resource name"=w772, "error in (no error)"=w771) -> ("VISA resource name out"=w766:refnum<visa-resource-name>, "error out"=w765:errorcluster)  [unwired: 12 in]
                }
              }
              frame #2 {
                n270 = local write "Realiza medição WT230"(FALSE ("Realiza medição")) -> ()
                n271 = property on="Realiza medição WT230" class="Bool (strict)"("DisabledEnum"=T23."Enabled" ("Disabled")) -> ()  [unwired: 2 in, 2 out]
              }
            }
          }
        }
        n272 = local read "stop geral"() -> (w753:bool)
      }
      n273 = while {
        stop <- w234 stop-if-true
        n274 = local read "Liga aquecedor"() -> (w235:bool)
        n275 = case shown="True" w235 {
          frame False {
            n276 = Wait (ms)(milliseconds to wait=u32 100) -> ()  [unwired: 1 out]
          }
          frame True {
            w241 = T33 0 items=["no dialog", "OK message", "continue or stop message", "OK message + warnings", "continue/stop + warnings"] ("type of dialog (OK msg:1)")
            w252 = 10123 items=["Finite Samples"=10178, "Continuous Samples"=10123, "Hardware Timed Single Point"=12522]  # Sample Mode
            n277 = call-poly <vilib>:"DAQmx Create Virtual Channel.vi"("frequency"="Frequency", "duty cycle"="Duty Cycle", "counter"=tag "Dev1/ctr0" ("Counter")) -> ("task out"=w255:refnum<k21>, "error out"=w254:errorcluster)  [unwired: 11 in]
            n278 = property class="DAQmx Channel"(reference=w255, error in=w254, "CO.Pulse.Term"=tag "/Dev1/PFI12" ("Output Terminal")) -> (reference out=w251:refnum<k21>, error out=w250:errorcluster)
            n279 = call-poly <vilib>:"DAQmx Timing.vi"("task/channels in"=w251, "sample mode"=w252, "error in"=w250) -> ("task out"=w249:refnum<k21>, "error out"=w248:errorcluster)  [unwired: 11 in]
            n280 = call <vilib>:"DAQmx Start Task.vi"("task/channels in"=w249, "error in"=w248) -> ("task out"=w247:refnum<k21>, "error out"=w246:errorcluster)  [unwired: 12 in]
            n281 = while {
              tunnel: w247 -> [w264]
              tunnel: w246 -> [w262]
              tunnel: [w273] -> w243
              tunnel: [w274] -> w244
              tunnel: [FALSE ("Liga aquecedor")] -> w240
              tunnel: "Duty Cycle" -> [w260]
              tunnel: "Frequency" -> [w257]
              stop <- w267 stop-if-true
              n282 = local read "Duty Cycle"() -> (w258:dbl)
              n283 = Not Equal?(x=w260, y=w258) -> (x != y?=w259:bool)
              n284 = case shown="True" w259 {
                tunnel: [w276 w279] -> w263
                tunnel: w264 -> [w276 w280]
                tunnel: [w275 w281] -> w261
                tunnel: w262 -> [w275 w282]
                tunnel: w258 -> [_ w278]
                tunnel: w257 -> [_ w277]
                frame False {
                }
                frame True {
                  n285 = call-poly <vilib>:"DAQmx Write.vi"("task/channels in"=w280, "frequency"=w277, "duty cycle"=w278, "error in"=w282) -> ("task out"=w279:refnum<k21>, "error out"=w281:errorcluster)  [unwired: 9 in, 1 out]
                }
              }
              n286 = local read "Liga aquecedor"() -> (w270:bool)
              n287 = call <vilib>:"DAQmx Is Task Done.vi"("task/channels in"=w263, "error in"=w261) -> ("task out"=w274:refnum<k21>, "error out"=w273:errorcluster)  [unwired: 11 in, 1 out]
              n288 = local read "stop geral"() -> (w265:bool)
              n289 = Unbundle By Name(w273) -> ("status"=w272:bool)
              n290 = Not(x=w270) -> (.not. x?=w268:bool)
              n291 = Or(x=w272, y=w268) -> (x .or. y?=w266:bool)
              n292 = Or(x=w266, y=w265) -> (x .or. y?=w267:bool)
              n293 = Wait Until Next ms Multiple(millisecond multiple=u32 10) -> ()  [unwired: 1 out]
            }
            n294 = call <vilib>:"DAQmx Stop Task.vi"("task/channels in"=w244, "error in"=w243) -> ("task out"=w239:refnum<k21>, "error out"=w245:errorcluster)  [unwired: 12 in]
            n295 = local write "Liga aquecedor"(w240) -> ()
            n296 = call <vilib>:"DAQmx Clear Task.vi"("task in"=w239, "error in"=w245) -> ("error out"=w242:errorcluster)  [unwired: 13 in]
            n297 = call <vilib>:"Simple Error Handler.vi"("error code (no error:0)"=w241, "error in (no error)"=w242) -> ()  [unwired: 3 in, 5 out]
          }
        }
        n298 = local read "stop geral"() -> (w234:bool)
      }
      n299 = while {
        shift-right: [w657] -> _
        shift-left: 0.0 ("RPM encoder") -> [w656]
        stop <- w666 stop-if-true
        # "Aquisição - RPM"
        n300 = flat-sequence {
          tunnel: [w687] -> w676
          tunnel: [w692] -> w677
          tunnel: w676 -> [w692]
          tunnel: ["RPM Rate (Hz)"] -> w675
          tunnel: [w690] -> w671
          tunnel: [w689] -> w663
          tunnel: ["RPM Samples (n)"] -> w660
          tunnel: w677 -> [w694]
          tunnel: w663 -> [w693]
          tunnel: [w693] -> w662
          tunnel: [w693] -> w661
          frame #0 {
            n301 = local read "semaforo medição"() -> (w686:T11)
            n302 = call <vilib>:"Acquire Semaphore.vi"("semaphore"=w686) -> ("semaphore out"=w687:T11)  [unwired: 4 in, 2 out]
          }
          frame #1 {
            n303 = call "DAQ Assistant5"("rate"="RPM Rate (Hz)", "number of samples"="RPM Samples (n)") -> ("data"=w689:dynamicdata)  [unwired: 15 in, 2 out]
            n304 = call <vilib>:"High Resolution Relative Seconds.vi"() -> ("relative seconds"=w690:dbl)
          }
          frame #2 {
            n305 = call <vilib>:"Release Semaphore.vi"("semaphore"=w694) -> ()  [unwired: 5 in, 2 out]
          }
        }
        n306 = local read "Referência entrada (RPM)"() -> (w658:dbl)
        n307 = local read "Habilitar (RPM)"() -> (w659:bool)
        n308 = case shown="False" w659 {
          tunnel: [w681 w685] -> w669
          tunnel: [w681 w684] -> w668
          tunnel: [w681 w683] -> w667
          tunnel: [w680 w682] -> w664
          frame False {
            w681 = nan
            n309 = local read "Velocidade (RPM)"() -> (w680:u16)
          }
          frame True {
            n310 = local read "Referência entrada (RPM)"() -> (w685:dbl)
            n311 = local read "var controle rpm"() -> (w682:u16)
            n312 = local read "lim sup rpm"() -> (w684:dbl)
            n313 = local read "lim inf rpm"() -> (w683:dbl)
          }
        }
        n314 = Reciprocal(x=w675) -> (1/x=w674:dbl)
        n315 = call "Convert from Dynamic Data5"("Dynamic Data Type"=w662) -> ("Array"=w678:dbl[])  [unwired: 3 in]
        n316 = call "edge_count.vi"("Ultimo RPM encoder"=w656, "RPM setpoint"=w658, "malha controle?"=w659, "RPM Samples (n)"=w660, "1/rate"=w674, "Data"=w678) -> ("RPM encoder"=w657:dbl, "RPM"=w670:dbl)  [unwired: 4 in]
        "RPM" <- w670
        n317 = local read "Ensaiando?"() -> (w672:bool)
        n318 = Bundle("relative seconds"=w671, "RPM"=w670, "Referência entrada (RPM)"=w669, "lim sup rpm"=w668, "lim inf rpm"=w667, "var controle rpm"=w664) -> (→"rpm values cluster":T34)  [unwired: 1 in]
        n319 = Bundle("RPM"=w670, "Referência entrada (RPM)"=w669, "lim sup rpm"=w668, "lim inf rpm"=w667) -> (w673:T18)  [unwired: 1 in]
        n320 = case shown="False" w672 {
          tunnel: w673 -> [w679 _]
          frame False {
            "Chart RPM" <- w679
          }
          frame True {
          }
        }
        n321 = local read "stop geral"() -> (w666:bool)
        "Waveform RPM" <- w661
      }
      n322 = while {
        stop <- w93 stop-if-true
        # "Aquisição - Wattímetro PZ4000"
        n323 = local read "Realiza medição PZ4000"() -> (w92:bool)
        n324 = case shown="True" w92 {
          tunnel: T23."Disabled and Grayed Out" ("Disabled") -> [_ w97]
          frame False {
            n325 = Wait (ms)(milliseconds to wait=u32 100) -> ()  [unwired: 1 out]
          }
          frame True {
            n326 = property on="Realiza medição PZ4000" class="Bool (strict)"("DisabledEnum"=w97) -> ()  [unwired: 2 in, 2 out]
            n327 = local read "Waveform?"() -> (w99:bool)
            n328 = Or(x=w99, y=TRUE) -> (x .or. y?=w100:bool)
            n329 = case shown="True" w100 {
              tunnel: refnum<visa-resource-name> "PZ" ("VISA resource name") -> [w110 w162]
              tunnel: [w105 w163] -> w101
              tunnel: [T23."Enabled" ("Disabled") T23."Enabled" ("Disabled")] -> w96
              tunnel: [FALSE ("Realiza medição PZ4000") FALSE ("Realiza medição PZ4000")] -> w95
              frame False {
                n330 = call <instrlib>:"Start Stop.vi"("VISA resource name"=w110, "Start/Stop (F: Stop)"=TRUE) -> ("VISA resource name out"=w109:refnum<visa-resource-name>, "error out"=w108:errorcluster)  [unwired: 12 in]
                n331 = while {
                  tunnel: w109 -> [w121]
                  tunnel: w108 -> [w120]
                  tunnel: [w115] -> w107
                  tunnel: [w114] -> w106
                  stop <- w118 stop-if-true
                  w124 = u16 1 items=["", "Preset1", "Preset2", "Preset3", "Preset4"] ("Preset (1: Preset1)")
                  n332 = while {
                    tunnel: [w141] -> w126
                    tunnel: [w139] -> w127
                    tunnel: w120 -> [w138]
                    tunnel: w121 -> [w136]
                    tunnel: [w135] -> w128
                    shift-right: [w129] -> _
                    shift-left: TRUE ("Boolean") -> [w131]
                    stop <- w134 stop-if-true
                    n333 = call <instrlib>:"Query Condition Status.vi"("VISA resource name"=w136, "error in (no error)"=w138) -> ("VISA resource name out"=w141:refnum<visa-resource-name>, "Condition"=w137:i32, "error out"=w139:errorcluster)  [unwired: 11 in]
                    n334 = Wait (ms)(milliseconds to wait=u32 50) -> ()  [unwired: 1 out]
                    n335 = Not(x=w131) -> (.not. x?=w130:bool)
                    n336 = call "cond_status_translate.vi"("Condition"=w137) -> ("Boolean"=w129:bool)  [unwired: 9 in, 1 out]
                    n337 = local read "stop geral"() -> (w133:bool)
                    n338 = And(x=w130, y=w129) -> (x .and. y?=w132:bool)
                    n339 = call <vilib>:"High Resolution Relative Seconds.vi"() -> ("relative seconds"=w135:dbl)
                    n340 = Or(x=w132, y=w133) -> (x .or. y?=w134:bool)
                  }
                  n341 = local read "Ensaiando?"() -> (w122:bool)
                  n342 = call <instrlib>:"Read Numeric Normal.vi"("VISA resource name"=w126, "Preset (1: Preset 1)"=w124, "Number of Item (15)"=u16 30, "error in (no error)"=w127) -> ("VISA resource name out"=w115:refnum<visa-resource-name>, "Measure"=w125:dbl[], "error out"=w114:errorcluster)  [unwired: 8 in, 1 out]
                  n343 = call "power_clusterer.vi"("relative seconds"=w128, "Measure"=w125) -> ("Cluster"=w112:T4)  [unwired: 9 in]
                  "watt num cluster" <- w112
                  n344 = local read "Medição contínua? PZ4000"() -> (w117:bool)
                  n345 = case shown="False" w122 {
                    tunnel: w112 -> [w154 _]
                    frame False {
                      n346 = Unbundle By Name(w154) -> ("V(A)"=w159:dbl, "V(B)"=w158:dbl, "V(E)"=w153:dbl, "I(A)"=w152:dbl, "I(B)"=w151:dbl, "I(E)"=w150:dbl, "PC(A)"=w149:dbl, "PC(B)"=w148:dbl, "PC(T)"=w147:dbl, "PL(A)"=w146:dbl, "PL(B)"=w145:dbl, "PL(T)"=w144:dbl, "PC(E)"=w143:dbl, "PL(E)"=w142:dbl)
                      n347 = Bundle("PC(A)"=w149, "PC(B)"=w148, "PC(T)"=w147, "PL(A)"=w146, "PL(B)"=w145, "PL(T)"=w144, "PC(E)"=w143, "PL(E)"=w142) -> (→"Chart potencia numeric":T14)  [unwired: 1 in]
                      n348 = Bundle("I(A)"=w152, "I(B)"=w151, "I(E)"=w150) -> (→"Chart corrente numeric":cluster{"I(A)":dbl, "I(B)":dbl, "I(E)":dbl})  [unwired: 1 in]
                      n349 = Bundle("V(A)"=w159, "V(B)"=w158, "V(E)"=w153) -> (→"Chart tensão numeric":cluster{"V(A)":dbl, "V(B)":dbl, "V(E)":dbl})  [unwired: 1 in]
                    }
                    frame True {
                    }
                  }
                  n350 = local read "stop geral"() -> (w119:bool)
                  n351 = Not(x=w117) -> (.not. x?=w116:bool)
                  n352 = Or(x=w116, y=w119) -> (x .or. y?=w118:bool)
                }
                n353 = call <instrlib>:"Start Stop.vi"("VISA resource name"=w107, "error in (no error)"=w106) -> ("error out"=w105:errorcluster)  [unwired: 12 in, 1 out]
              }
              frame True {
                n354 = while {
                  tunnel: [w175] -> w163
                  tunnel: w162 -> [w168]
                  stop <- w171 stop-if-true
                  n355 = call <instrlib>:"Wait Update.vi"("VISA resource name"=w168) -> ("VISA resource name out"=w170:refnum<visa-resource-name>, "error out"=w169:errorcluster)  [unwired: 13 in]
                  n356 = while {
                    tunnel: [w222] -> w177
                    tunnel: [w220] -> w176
                    shift-right: [w213] -> _
                    shift-left: TRUE ("Boolean") -> [w217]
                    tunnel: w170 -> [w216]
                    tunnel: w169 -> [w215]
                    shift-right: [w208] -> _
                    shift-left: 0 -> [w209]
                    tunnel: [w201] -> w165
                    stop <- w202 stop-if-true
                    n357 = call <instrlib>:"Query Condition Status.vi"("VISA resource name"=w216, "error in (no error)"=w215) -> ("VISA resource name out"=w222:refnum<visa-resource-name>, "Condition"=w219:i32, "error out"=w220:errorcluster)  [unwired: 11 in]
                    n358 = Wait (ms)(milliseconds to wait=u32 50) -> ()  [unwired: 1 out]
                    n359 = Not(x=w217) -> (.not. x?=w214:bool)
                    n360 = call "cond_status_translate.vi"("Condition"=w219) -> ("Boolean"=w212:bool, "Boolean 2"=w211:bool)  [unwired: 9 in]
                    n361 = Or(x=w212, y=w211) -> (x .or. y?=w210:bool)
                    n362 = Select(t=w214, s=w212, f=w212) -> (s? t:f=w213:bool)
                    n363 = local read "stop geral"() -> (w218:bool)
                    n364 = And(x=w214, y=w210) -> (x .and. y?=w203:bool)
                    n365 = case shown="False" w203 {
                      tunnel: w209 -> [w224 w225]
                      tunnel: [w223 w225] -> w208
                      frame False {
                        n366 = Increment(x=w224) -> (x+1=w223:i32)
                      }
                      frame True {
                      }
                    }
                    n367 = Greater Or Equal?(x=w208, y=100) -> (x >= y?=w206:bool)
                    n368 = Select(t=TRUE ("Boolean"), s=w206, f=w203) -> (s? t:f=w204:bool)
                    n369 = Or(x=w204, y=w218) -> (x .or. y?=w202:bool)
                    n370 = call <vilib>:"High Resolution Relative Seconds.vi"() -> ("relative seconds"=w201:dbl)
                  }
                  n371 = for {
                    N: 6 -> [_]
                    tunnel: [w194] -> w183 mode=indexing
                    shift-right: [w192] -> _
                    shift-left: w177 -> [w190]
                    shift-right: [w191] -> w175
                    shift-left: w176 -> [w187]
                    i -> [w195]
                    stop <- w193 stop-if-true
                    w185 = u32 0 ("Start Point (0)")
                    w184 = u32 100000 ("End Point (1000)")
                    n372 = Increment(x=w195) -> (x+1=w186:i32)
                    n373 = call <instrlib>:"Config Waveform.vi"("VISA resource name"=w190, "End Point (1000)"=w184, "Start Point (0)"=w185, "Select Trace (1)"=w186, "error in (no error)"=w187) -> ("VISA resource name out"=w189:refnum<visa-resource-name>, "error out"=w188:errorcluster)  [unwired: 9 in]
                    n374 = To Unsigned Word Integer(number=w186) -> (unsigned 16bit integer=w196:u16)
                    n375 = call <instrlib>:"Read Range.vi"("VISA resource name"=w189, "error in (no error)"=w188) -> ("VISA resource name out"=w200:refnum<visa-resource-name>, "Range"=w197:dbl, "error out"=w199:errorcluster)  [unwired: 11 in]
                    n376 = call <instrlib>:"Read Waveform.vi"("VISA resource name"=w200, "End Point (1000)"=w184, "Start Point (0)"=w185, "Select Trace (1)"=w196, "error in (no error)"=w199) -> ("VISA resource name out"=w192:refnum<visa-resource-name>, "Waveform Data"=w198:string, "error out"=w191:errorcluster)  [unwired: 8 in]
                    n377 = local read "stop geral"() -> (w193:bool)
                    n378 = call <instrlib>:"Waveform Data Convert.vi"("Input Data"=w198, "Range"=w197) -> ("Output"=w194:dbl[])  [unwired: 11 in, 2 out]
                  }
                  n379 = local read "Medição contínua? PZ4000"() -> (w173:bool)
                  n380 = local read "stop geral"() -> (w174:bool)
                  n381 = Not(x=w173) -> (.not. x?=w172:bool)
                  n382 = Or(x=w172, y=w174) -> (x .or. y?=w171:bool)
                  n383 = call "waveform_demux.vi"("t"=w165, "dt integracao"="dt integracao", "Output"=w183) -> ("watt num cluster"=w164:T4, "Array"=→"Corrente":dbl[][], "output cluster"=→"Chart Potencia":cluster{dbl, dbl, dbl, dbl}, "Array 2"=→"Tensão":dbl[][])  [unwired: 5 in]
                  n384 = local write "watt num cluster"(w164) -> ()
                }
              }
            }
            "error out" <- w101
            n385 = local write "Realiza medição PZ4000"(w95) -> ()
            n386 = property on="Realiza medição PZ4000" class="Bool (strict)"("DisabledEnum"=w96) -> ()  [unwired: 2 in, 2 out]
          }
        }
        n387 = local read "stop geral"() -> (w93:bool)
      }
      n388 = while {
        stop <- w76 stop-if-true
        n389 = local read "stop geral"() -> (w76:bool)
        n390 = local read "Salvar encoder"() -> (w75:bool)
        n391 = case shown="True" w75 {
          frame False {
            n392 = Wait (ms)(milliseconds to wait=u32 100 ("millisecond multiple")) -> ()  [unwired: 1 out]
          }
          frame True {
            n393 = for {
              N: "encoder files" -> [_]
              tunnel: [FALSE ("Salvar encoder")] -> w84
              tunnel: [w86] -> w80 mode=indexing
              i -> [w90]
              n394 = local read "Waveform RPM"() -> (w87:dynamicdata)
              n395 = Wait (ms)(milliseconds to wait="encoder wait") -> ()  [unwired: 1 out]
              n396 = call "Convert from Dynamic Data2"("Dynamic Data Type"=w87) -> ("Array"=w86:dbl[])  [unwired: 3 in]
              "encoder saved" <- w90
            }
            n397 = local write "Salvar encoder"(w84) -> ()
            n398 = Transpose 2D Array(2D array=w80) -> (transposed array=w81:dbl[][])
            n399 = call "File Dialog"("start path"=path "C:/Users/zomer/Desktop/zomer/LabVIEW/dyna_liae/encoder artigo") -> ("selected path"=w78:path)  [unwired: 11 in, 3 out]
            n400 = Array To Spreadsheet String(array=w81, 3:"%g" ("format string")) -> (spreadsheet string=w83:string)  [unwired: 1 in]
            n401 = Write to Text File(file (use dialog)=w78, text=w83) -> ()  [unwired: 2 in, 3 out]
          }
        }
      }
      n402 = while {
        stop <- w596 stop-if-true
        # "Controle de Torque"
        n403 = local read "stop geral"() -> (w598:bool)
        n404 = local read "Habilitar (Torque)"() -> (w600:bool)
        n405 = Not(x=w598) -> (.not. x?=w599:bool)
        n406 = And(x=w600, y=w599) -> (x .and. y?=w597:bool)
        n407 = case shown="True" w597 {
          frame False {
            n408 = Wait (ms)(milliseconds to wait=u32 100) -> ()  [unwired: 1 out]
          }
          frame True {
            n409 = flat-sequence {
              tunnel: [w608] -> w605
              tunnel: [w606] -> w602
              tunnel: w605 -> [w615]
              tunnel: [w615] -> w604
              tunnel: [w613] -> w603
              tunnel: w602 -> [w613]
              tunnel: w604 -> [w622]
              tunnel: w603 -> [w619]
              frame #0 {
                n410 = call <instrlib>:"GENie Config Voltage Limit.vi"("Volt Limit"=18.0, "VISA"=refnum<visa-resource-name> "Lambda" ("VISA name")) -> ("error out"=w607:errorcluster, "VISA out"=w612:refnum<visa-resource-name>)  [unwired: 8 in]
                n411 = call <instrlib>:"GENie Config Current Limit.vi"("error"=w607, "Current Limit"=0.0, "VISA"=w612) -> ("error out"=w606:errorcluster, "VISA out"=w608:refnum<visa-resource-name>)  [unwired: 7 in]
              }
              frame #1 {
                n412 = property on="Liga saída" class="Bool (strict)"("Val(Sgnl)"=TRUE ("Value (Signaling)")) -> ()  [unwired: 2 in, 2 out]
              }
              frame #2 {
                n413 = while {
                  tunnel: [w642] -> w624
                  tunnel: [0.0 ("Current Limit")] -> w625
                  tunnel: w622 -> [w640]
                  tunnel: [w635] -> w621
                  tunnel: [FALSE ("Value (Signaling)")] -> w620
                  tunnel: w619 -> [w633]
                  tunnel: [w632] -> w618
                  shift-right: [FALSE ("reinitialize? (F)")] -> _
                  shift-left: TRUE ("reinitialize? (F)") -> [w631]
                  stop <- w637 stop-if-true
                  n414 = local read "torque mean"() -> (w629:dbl)
                  n415 = local read "Referência entrada (mN.m)"() -> (w646:dbl)
                  n416 = Wait (ms)(milliseconds to wait=u32 500) -> ()  [unwired: 1 out]
                  n417 = disable-structure shown="Enabled" {
                    disable-tunnel: ["PID Torque" w653] -> w641
                    disable-tunnel: w629 -> [_ w652]
                    frame Disabled {
                    }
                    frame Enabled {
                      n418 = call-poly <vilib>:"PID Gain Schedule.vi"("PID gain schedule"="PID gain schedule", "gain scheduling value"=w652) -> ("PID gains out"=w653:T20)  [unwired: 2 in, 1 out]
                    }
                  }
                  n419 = local read "Habilitar (Torque)"() -> (w650:bool)
                  n420 = local read "stop geral"() -> (w648:bool)
                  n421 = local read "RPM"() -> (w639:dbl)
                  n422 = Not(x=w650) -> (.not. x?=w649:bool)
                  n423 = call-poly <vilib>:"PID.vi"("reinitialize? (F)"=w631, "output range"=cluster{"output high":dbl, "output low":dbl} {"output high"=0.4, "output low"=0.0}, "dt (s)"=0.2, "PID gains"=w641, "process variable"=w629, "setpoint"=w646) -> ("output"=w643:dbl)  [unwired: 4 in, 1 out]
                  "var controle torque" <- w643
                  n424 = Or(x=w648, y=w649) -> (x .or. y?=w638:bool)
                  n425 = Equal To 0?(x=w639) -> (x = 0?=w635:bool)
                  n426 = Or(x=w635, y=w638) -> (x .or. y?=w637:bool)
                  n427 = call <instrlib>:"GENie Config Current Limit.vi"("error"=w633, "Current Limit"=w643, "VISA"=w640) -> ("error out"=w632:errorcluster, "VISA out"=w642:refnum<visa-resource-name>)  [unwired: 7 in]
                }
                n428 = case shown="True" w621 {
                  frame False {
                  }
                  frame True {
                    n429 = local read "Parâmetros serial"() -> (w628:T22)
                    n430 = call "Serial_control.vi"("Enviar número"=u16 0, "Função"=T26."Set Speed", "comm cluster"=w628) -> ()  [unwired: 2 in, 4 out]
                  }
                }
                n431 = call <instrlib>:"GENie Config Current Limit.vi"("error"=w618, "Current Limit"=0.0, "VISA"=w624) -> ("error out"=→"error out 2":errorcluster)  [unwired: 7 in, 1 out]
                n432 = local write "Referência entrada (mN.m)"(w625) -> ()
                n433 = property on="Habilitar (Torque)" class="Bool (strict)"("Val(Sgnl)"=w620) -> ()  [unwired: 2 in, 2 out]
              }
              frame #3 {
                n434 = property on="Liga saída" class="Bool (strict)"("Val(Sgnl)"=FALSE ("Value (Signaling)")) -> ()  [unwired: 2 in, 2 out]
              }
            }
          }
        }
        n435 = local read "stop geral"() -> (w596:bool)
      }
      n436 = while {
        stop <- w699 stop-if-true
        # "RP - RPM"
        n437 = local read "stop geral"() -> (w696:bool)
        n438 = local read "Habilitar (RPM)"() -> (w698:bool)
        n439 = Not(x=w696) -> (.not. x?=w697:bool)
        n440 = And(x=w698, y=w697) -> (x .and. y?=w695:bool)
        n441 = case shown="True" w695 {
          selector: w695 -> [w700 _]
          frame False {
            n442 = local write "rpm em rp?"(w700) -> ()
          }
          frame True {
            n443 = while {
              shift-right: [w715] -> _
              shift-left: 0 -> [w717]
              stop <- w710 stop-if-true
              n444 = local read "Margem RPM (%)"() -> (w709:dbl)
              n445 = local read "Habilitar (RPM)"() -> (w713:bool)
              n446 = Wait (ms)(milliseconds to wait=u32 200) -> ()  [unwired: 1 out]
              n447 = local read "stop geral"() -> (w711:bool)
              n448 = local read "Referência entrada (RPM)"() -> (w718:dbl)
              n449 = Not(x=w713) -> (.not. x?=w712:bool)
              n450 = Divide(x=w709, y=100.0) -> (x/y=w707:dbl)
              n451 = Or(x=w711, y=w712) -> (x .or. y?=w710:bool)
              n452 = Increment(x=w707) -> (x+1=w705:dbl)
              n453 = Decrement(x=w707) -> (x-1=w708:dbl)
              n454 = Absolute Value(x=w708) -> (abs(x)=w704:dbl)
              n455 = Increment(x=w717) -> (x+1=w721:i32)
              n456 = Multiply(x=w705, y=w718) -> (x*y=w703:dbl)
              "lim sup rpm" <- w703
              n457 = Multiply(x=w704, y=w718) -> (x*y=w702:dbl)
              "lim inf rpm" <- w702
              n458 = local read "RPM"() -> (w719:dbl)
              n459 = In Range and Coerce(upper limit=w703, x=w719, lower limit=w702) -> (In Range?=w722:bool)  [unwired: 1 out]
              n460 = Select(t=w721, s=w722, f=0) -> (s? t:f=w715:i32)
              n461 = Greater Or Equal?(x=w715, y=20) -> (x >= y?=→"rpm em rp?":bool)
            }
          }
        }
        n462 = local read "stop geral"() -> (w699:bool)
      }
      n463 = while {
        stop <- w728 stop-if-true
        # "RP - Torque"
        n464 = local read "stop geral"() -> (w727:bool)
        n465 = local read "Habilitar (Torque)"() -> (w725:bool)
        n466 = Not(x=w727) -> (.not. x?=w726:bool)
        n467 = And(x=w725, y=w726) -> (x .and. y?=w724:bool)
        n468 = case shown="True" w724 {
          selector: w724 -> [w729 _]
          frame False {
            n469 = local write "torque em rp?"(w729) -> ()
          }
          frame True {
            n470 = while {
              shift-right: [w746] -> _
              shift-left: 0 -> [w747]
              stop <- w739 stop-if-true
              n471 = local read "Margem torque (%)"() -> (w736:dbl)
              n472 = local read "Habilitar (Torque)"() -> (w742:bool)
              n473 = Wait (ms)(milliseconds to wait=u32 200) -> ()  [unwired: 1 out]
              n474 = local read "stop geral"() -> (w740:bool)
              n475 = local read "Referência entrada (mN.m)"() -> (w752:dbl)
              n476 = Not(x=w742) -> (.not. x?=w741:bool)
              n477 = Divide(x=w736, y=100.0) -> (x/y=w738:dbl)
              n478 = Or(x=w740, y=w741) -> (x .or. y?=w739:bool)
              n479 = Increment(x=w738) -> (x+1=w734:dbl)
              n480 = Decrement(x=w738) -> (x-1=w737:dbl)
              n481 = local read "torque mean"() -> (w751:dbl)
              n482 = Absolute Value(x=w737) -> (abs(x)=w733:dbl)
              n483 = Increment(x=w747) -> (x+1=w749:i32)
              n484 = Multiply(x=w734, y=w752) -> (x*y=w732:dbl)
              "lim sup torque" <- w732
              n485 = Multiply(x=w733, y=w752) -> (x*y=w731:dbl)
              "lim inf torque" <- w731
              n486 = In Range and Coerce(upper limit=w732, x=w751, lower limit=w731) -> (In Range?=w748:bool)  [unwired: 1 out]
              n487 = Select(t=w749, s=w748, f=0) -> (s? t:f=w746:i32)
              n488 = Greater Or Equal?(x=w746, y=20) -> (x >= y?=→"torque em rp?":bool)
            }
          }
        }
        n489 = local read "stop geral"() -> (w728:bool)
      }
      n490 = while {
        stop <- w881 stop-if-true
        # "Controle de Velocidade Angular"
        n491 = local read "stop geral"() -> (w880:bool)
        n492 = local read "Habilitar (RPM)"() -> (w878:bool)
        n493 = Not(x=w880) -> (.not. x?=w879:bool)
        n494 = And(x=w878, y=w879) -> (x .and. y?=w877:bool)
        n495 = case shown="True" w877 {
          frame False {
            n496 = Wait (ms)(milliseconds to wait=u32 100) -> ()  [unwired: 1 out]
          }
          frame True {
            n497 = while {
              tunnel: [w889] -> w885
              shift-right: [FALSE ("reinitialize? (F)")] -> _
              shift-left: TRUE ("reinitialize? (F)") -> [w887]
              stop <- w893 stop-if-true
              n498 = local read "Referência entrada (RPM)"() -> (w891:dbl)
              n499 = local read "Habilitar (RPM)"() -> (w896:bool)
              n500 = Wait (ms)(milliseconds to wait=u32 500) -> ()  [unwired: 1 out]
              n501 = local read "stop geral"() -> (w894:bool)
              n502 = Not(x=w896) -> (.not. x?=w895:bool)
              n503 = Or(x=w894, y=w895) -> (x .or. y?=w893:bool)
              n504 = Equal To 0?(x=w891) -> (x = 0?=w890:bool)
              n505 = case shown="False" w890 {
                tunnel: w891 -> [w902 _]
                tunnel: [w901 w908] -> w889
                tunnel: w887 -> [w900 _]
                frame False {
                  n506 = local read "RPM"() -> (w905:dbl)
                  n507 = local read "Parâmetros serial"() -> (w901:T22)
                  n508 = call-poly <vilib>:"PID.vi"("reinitialize? (F)"=w900, "output range"=cluster{"output high":dbl, "output low":dbl} {"output high"=5050.0, "output low"=1000.0}, "dt (s)"=0.5, "PID gains"="PID RPM", "process variable"=w905, "setpoint"=w902) -> ("output"=w899:dbl)  [unwired: 4 in, 1 out]
                  n509 = To Unsigned Word Integer(number=w899) -> (unsigned 16bit integer=w897:u16)
                  "var controle rpm" <- w897
                  n510 = call "Serial_control.vi"("Enviar número"=w897, "Função"=T26."Set Speed", "comm cluster"=w901) -> ("Error Out"=→"Error Out":T1)  [unwired: 2 in, 3 out]
                }
                frame True {
                  n511 = local read "Parâmetros serial"() -> (w908:T22)
                }
              }
            }
            n512 = call "Serial_control.vi"("Enviar número"=u16 0, "Função"=T26."Set Speed", "comm cluster"=w885) -> ()  [unwired: 2 in, 4 out]
          }
        }
        n513 = local read "stop geral"() -> (w881:bool)
      }
      n514 = while {
        shift-right: [w439] -> _
        shift-left: w71 -> [w447]
        shift-right: [w433] -> _
        shift-left: 0.0 ("mean") -> [w416]
        shift-right: [w438] -> _
        shift-left: w71 -> [w446]
        shift-right: [w437] -> _
        shift-left: w71 -> [w445]
        shift-right: [w436] -> _
        shift-left: w71 -> [w444]
        shift-right: [w435] -> _
        shift-left: w71 -> [w443]
        shift-right: [w425] -> _
        shift-left: 0.0 ("mean") -> [w341]
        shift-right: [w421] -> _
        shift-left: w68 -> [w431]
        shift-right: [w420] -> _
        shift-left: w68 -> [w430]
        shift-right: [w419] -> _
        shift-left: w68 -> [w429]
        shift-right: [w418] -> _
        shift-left: w68 -> [w428]
        shift-right: [w417] -> _
        shift-left: w68 -> [w427]
        shift-right: [w399] -> _
        shift-left: 0.0 ("mean") -> [w340]
        shift-right: [w398] -> _
        shift-left: w66 -> [w414]
        shift-right: [w397] -> _
        shift-left: w66 -> [w413]
        shift-right: [w396] -> _
        shift-left: w66 -> [w412]
        shift-right: [w395] -> _
        shift-left: w66 -> [w411]
        shift-right: [w369] -> _
        shift-left: w66 -> [w407]
        shift-right: [w368] -> _
        shift-left: w66 -> [w410]
        shift-right: [w394] -> _
        shift-left: w66 -> [w409]
        shift-right: [w393] -> _
        shift-left: w66 -> [w408]
        shift-right: [w371] -> _
        shift-left: w68 -> [w375]
        shift-right: [w376] -> _
        shift-left: w71 -> [w380]
        shift-right: [w350] -> _
        shift-left: w66 -> [w364]
        shift-right: [w349] -> _
        shift-left: w66 -> [w363]
        shift-right: [w348] -> _
        shift-left: w66 -> [w362]
        shift-right: [w347] -> _
        shift-left: w66 -> [w361]
        shift-right: [w346] -> _
        shift-left: w66 -> [w360]
        shift-right: [w352] -> _
        shift-left: w66 -> [w367]
        shift-right: [w351] -> _
        shift-left: w66 -> [w365]
        shift-right: [w338] -> _
        shift-left: 0.0 ("mean") -> [w339]
        shift-right: [w329] -> _
        shift-left: w63 -> [w337]
        shift-right: [w328] -> _
        shift-left: w63 -> [w336]
        shift-right: [w327] -> _
        shift-left: w63 -> [w335]
        shift-right: [w326] -> _
        shift-left: w63 -> [w334]
        shift-right: [w321] -> _
        shift-left: w63 -> [w325]
        shift-right: [w320] -> _
        shift-left: w63 -> [w324]
        shift-right: [w313] -> _
        shift-left: w63 -> [w317]
        shift-right: [w312] -> _
        shift-left: w63 -> [w316]
        stop <- w450 stop-if-true
        # "Baita loop de tratamento de dados, maior decepção da minha vida"
        n515 = local read "rpm values cluster"() -> (w432:T7)
        n516 = local read "watt num cluster"() -> (w415:T4)
        n517 = local read "temperature num cluster"() -> (w345:T3)
        n518 = Wait (ms)(milliseconds to wait=u32 50) -> ()  [unwired: 1 out]
        n519 = Unbundle By Name(w432) -> ("relative seconds"=w385:dbl, "RPM"=w426:dbl, "Referência entrada (RPM)"=w424:dbl, "lim sup rpm"=w423:dbl, "lim inf rpm"=w422:dbl, "var controle rpm"=w374:dbl)
        n520 = local read "torque values cluster"() -> (w448:T8)
        n521 = Unbundle By Name(w345) -> ("tempo"=w333:dbl, "t1 bobina"=w332:dbl, "t2 bobina"=w331:dbl, "t freio"=w330:dbl, "t rola tras"=w323:dbl, "t rola frente"=w322:dbl, "t amb"=w315:dbl, "duty cycle"=w314:dbl)
        n522 = Unbundle By Name(w415) -> ("V(A)"=w400:dbl, "I(A)"=w401:dbl, "V(B)"=w402:dbl, "I(B)"=w403:dbl, "PC(A)"=w404:dbl, "PC(B)"=w405:dbl, "PC(T)"=w406:dbl, "t"=w381:dbl, "PL(A)"=w366:dbl, "PL(B)"=w359:dbl, "PL(T)"=w358:dbl, "V(E)"=w357:dbl, "I(E)"=w356:dbl, "PC(E)"=w355:dbl, "PL(E)"=w354:dbl)
        n523 = Unbundle By Name(w448) -> ("relative seconds"=w392:dbl, "mean"=w434:dbl, "Referência entrada (mN.m)"=w442:dbl, "lim sup torque"=w441:dbl, "lim inf torque"=w440:dbl, "var controle torque"=w379:dbl)
        n524 = Equal?(x=w333, y=w339) -> (x = y?=w343:bool)
        n525 = Not A Number/Path/Refnum?(number/path/refnum=w333) -> (NaN/Path/Refnum?=w344:bool)
        n526 = Equal?(x=w385, y=w341) -> (x = y?=w387:bool)
        n527 = Equal?(x=w381, y=w340) -> (x = y?=w383:bool)
        n528 = Not A Number/Path/Refnum?(number/path/refnum=w385) -> (NaN/Path/Refnum?=w388:bool)
        n529 = Not A Number/Path/Refnum?(number/path/refnum=w381) -> (NaN/Path/Refnum?=w384:bool)
        n530 = Or(x=w344, y=w343) -> (x .or. y?=w342:bool)
        n531 = Equal?(x=w392, y=w416) -> (x = y?=w390:bool)
        n532 = Not A Number/Path/Refnum?(number/path/refnum=w392) -> (NaN/Path/Refnum?=w389:bool)
        n533 = Or(x=w388, y=w387) -> (x .or. y?=w386:bool)
        n534 = Or(x=w384, y=w383) -> (x .or. y?=w382:bool)
        n535 = Or(x=w390, y=w389) -> (x .or. y?=w391:bool)
        n536 = case shown="True" w342 {
          tunnel: w339 -> [_ w484]
          tunnel: [w475 w484] -> w338
          tunnel: w333 -> [w475 _]
          tunnel: w337 -> [w474 w483]
          tunnel: w336 -> [w472 w482]
          tunnel: w335 -> [w470 w481]
          tunnel: w334 -> [w467 w480]
          tunnel: [w473 w483] -> w329
          tunnel: [w471 w482] -> w328
          tunnel: [w469 w481] -> w327
          tunnel: [w466 w480] -> w326
          tunnel: w333 -> [w468 _]
          tunnel: w332 -> [w465 _]
          tunnel: w331 -> [w464 _]
          tunnel: w330 -> [w463 _]
          tunnel: [w462 w479] -> w321
          tunnel: [w461 w478] -> w320
          tunnel: w325 -> [w460 w479]
          tunnel: w324 -> [w459 w478]
          tunnel: w323 -> [w458 _]
          tunnel: w322 -> [w457 _]
          tunnel: w317 -> [w456 w477]
          tunnel: w316 -> [w455 w476]
          tunnel: w315 -> [w454 _]
          tunnel: w314 -> [w453 _]
          tunnel: [w452 w477] -> w313
          tunnel: [w451 w476] -> w312
          frame False {
            n537 = Build Array (concatenate)(w456, w454) -> (w452:dbl[])
            n538 = Build Array (concatenate)(w455, w453) -> (w451:dbl[])
            n539 = Build Array (concatenate)(w460, w458) -> (w462:dbl[])
            n540 = Build Array (concatenate)(w474, w468) -> (w473:dbl[])
            n541 = Build Array (concatenate)(w472, w465) -> (w471:dbl[])
            n542 = Build Array (concatenate)(w470, w464) -> (w469:dbl[])
            n543 = Build Array (concatenate)(w467, w463) -> (w466:dbl[])
            n544 = Build Array (concatenate)(w459, w457) -> (w461:dbl[])
          }
          frame True {
          }
        }
        n545 = case shown="False" w386 {
          tunnel: [w563 w569] -> w421
          tunnel: [w562 w568] -> w420
          tunnel: [w561 w567] -> w419
          tunnel: [w560 w566] -> w418
          tunnel: [w559 w565] -> w417
          tunnel: w341 -> [_ w570]
          tunnel: w431 -> [w558 w569]
          tunnel: w430 -> [w557 w568]
          tunnel: w429 -> [w556 w567]
          tunnel: w428 -> [w555 w566]
          tunnel: w427 -> [w554 w565]
          tunnel: [w549 w570] -> w425
          tunnel: w426 -> [w553 _]
          tunnel: w385 -> [w549 _]
          tunnel: w424 -> [w552 _]
          tunnel: w423 -> [w551 _]
          tunnel: w422 -> [w550 _]
          tunnel: w375 -> [w548 w564]
          tunnel: w374 -> [w547 _]
          tunnel: [w546 w564] -> w371
          frame False {
            n546 = Build Array (concatenate)(w558, w549) -> (w563:dbl[])
            n547 = Build Array (concatenate)(w557, w553) -> (w562:dbl[])
            n548 = Build Array (concatenate)(w556, w552) -> (w561:dbl[])
            n549 = Build Array (concatenate)(w555, w551) -> (w560:dbl[])
            n550 = Build Array (concatenate)(w554, w550) -> (w559:dbl[])
            n551 = Build Array (concatenate)(w548, w547) -> (w546:dbl[])
          }
          frame True {
          }
        }
        n552 = case shown="False" w382 {
          tunnel: w414 -> [w529 w545]
          tunnel: w413 -> [w528 w544]
          tunnel: w412 -> [w527 w543]
          tunnel: w411 -> [w526 w542]
          tunnel: w407 -> [w525 w541]
          tunnel: w410 -> [w524 w540]
          tunnel: w409 -> [w523 w539]
          tunnel: w408 -> [w522 w538]
          tunnel: [w514 w545] -> w398
          tunnel: [w513 w544] -> w397
          tunnel: [w512 w543] -> w396
          tunnel: [w511 w542] -> w395
          tunnel: [w510 w541] -> w369
          tunnel: [w509 w540] -> w368
          tunnel: [w508 w539] -> w394
          tunnel: [w507 w538] -> w393
          tunnel: w381 -> [w506 _]
          tunnel: w406 -> [w521 _]
          tunnel: w405 -> [w520 _]
          tunnel: w404 -> [w519 _]
          tunnel: w403 -> [w518 _]
          tunnel: w402 -> [w517 _]
          tunnel: w401 -> [w516 _]
          tunnel: w400 -> [w515 _]
          tunnel: [w506 w537] -> w399
          tunnel: w340 -> [_ w537]
          tunnel: w367 -> [w505 w536]
          tunnel: w366 -> [w504 _]
          tunnel: w365 -> [w503 w535]
          tunnel: w364 -> [w502 w534]
          tunnel: w363 -> [w501 w533]
          tunnel: w362 -> [w500 w532]
          tunnel: w361 -> [w499 w531]
          tunnel: w360 -> [w498 w530]
          tunnel: w359 -> [w497 _]
          tunnel: w358 -> [w496 _]
          tunnel: w357 -> [w495 _]
          tunnel: w356 -> [w494 _]
          tunnel: w355 -> [w493 _]
          tunnel: w354 -> [w492 _]
          tunnel: [w491 w536] -> w352
          tunnel: [w490 w535] -> w351
          tunnel: [w489 w534] -> w350
          tunnel: [w488 w533] -> w349
          tunnel: [w487 w532] -> w348
          tunnel: [w486 w531] -> w347
          tunnel: [w485 w530] -> w346
          frame False {
            n553 = Build Array (concatenate)(w505, w504) -> (w491:dbl[])
            n554 = Build Array (concatenate)(w503, w497) -> (w490:dbl[])
            n555 = Build Array (concatenate)(w502, w496) -> (w489:dbl[])
            n556 = Build Array (concatenate)(w501, w495) -> (w488:dbl[])
            n557 = Build Array (concatenate)(w500, w494) -> (w487:dbl[])
            n558 = Build Array (concatenate)(w499, w493) -> (w486:dbl[])
            n559 = Build Array (concatenate)(w498, w492) -> (w485:dbl[])
            n560 = Build Array (concatenate)(w529, w515) -> (w514:dbl[])
            n561 = Build Array (concatenate)(w528, w516) -> (w513:dbl[])
            n562 = Build Array (concatenate)(w527, w517) -> (w512:dbl[])
            n563 = Build Array (concatenate)(w526, w518) -> (w511:dbl[])
            n564 = Build Array (concatenate)(w525, w519) -> (w510:dbl[])
            n565 = Build Array (concatenate)(w524, w520) -> (w509:dbl[])
            n566 = Build Array (concatenate)(w523, w521) -> (w508:dbl[])
            n567 = Build Array (concatenate)(w522, w506) -> (w507:dbl[])
          }
          frame True {
          }
        }
        n568 = case shown="False" w391 {
          tunnel: [w588 w595] -> w439
          tunnel: [w587 w594] -> w438
          tunnel: [w586 w593] -> w437
          tunnel: [w585 w592] -> w436
          tunnel: [w574 w591] -> w435
          tunnel: w447 -> [w584 w595]
          tunnel: w446 -> [w583 w594]
          tunnel: w445 -> [w582 w593]
          tunnel: w444 -> [w581 w592]
          tunnel: w443 -> [w580 w591]
          tunnel: w392 -> [w575 _]
          tunnel: w434 -> [w576 _]
          tunnel: w442 -> [w579 _]
          tunnel: w441 -> [w578 _]
          tunnel: w440 -> [w577 _]
          tunnel: [w575 w590] -> w433
          tunnel: w416 -> [_ w590]
          tunnel: w380 -> [w573 w589]
          tunnel: [w572 w589] -> w376
          tunnel: w379 -> [w571 _]
          frame False {
            n569 = Build Array (concatenate)(w584, w575) -> (w588:dbl[])
            n570 = Build Array (concatenate)(w583, w576) -> (w587:dbl[])
            n571 = Build Array (concatenate)(w582, w579) -> (w586:dbl[])
            n572 = Build Array (concatenate)(w581, w578) -> (w585:dbl[])
            n573 = Build Array (concatenate)(w580, w577) -> (w574:dbl[])
            n574 = Build Array (concatenate)(w573, w571) -> (w572:dbl[])
          }
          frame True {
          }
        }
        n575 = Bundle By Name(cluster=T5 {"t"=[], "V(A)"=[], "I(A)"=[], "V(B)"=[], "I(B)"=[], "PC(A)"=[], "PC(B)"=[], "PC(T)"=[], "PL(T)"=[], "PL(B)"=[], "PL(A)"=[], "V(E)"=[], "PL(E)"=[], "PC(E)"=[], "I(E)"=[]} ("watt array cluster"), "V(A)"=w398, "I(A)"=w397, "V(B)"=w396, "I(B)"=w395, "PC(A)"=w369, "PC(B)"=w368, "PC(T)"=w394, "t"=w393, "PL(A)"=w352, "PL(B)"=w351, "PL(T)"=w350, "V(E)"=w349, "I(E)"=w348, "PC(E)"=w347, "PL(E)"=w346) -> (→"watt array cluster":T5)
        n576 = Bundle By Name(cluster=T6 {"t"=array[506 elements], "rpm"=array[506 elements], "ref"=array[506 elements], "lim sup"=array[506 elements], "lim inf"=array[506 elements], "var contr"=array[506 elements]} ("rpm array cluster"), "t"=w421, "rpm"=w420, "ref"=w419, "lim sup"=w418, "lim inf"=w417, "var contr"=w371) -> (→"rpm array cluster":T6)
        n577 = Bundle By Name(cluster=T2 {"t"=[6044.3009041, 7715.027126999999, 7720.028396899999, 7725.0284959, 7730.0286268, 7735.0287567, 7740.027851999999, 7745.0279567, 7750.028104399999, 7755.0281981], "t1 bobina"=[24.959, 25.151, 25.147, 25.147, 25.147, 25.145, 25.146, 25.146, 25.143, 25.144], "t2 bobina"=[25.008, 25.064, 25.063, 25.062, 25.062, 25.062, 25.062, 25.06, 25.059, 25.062], "t freio"=[24.495, 24.289, 24.29, 24.29, 24.295, 24.298, 24.295, 24.293, 24.294, 24.294], "t rola frente"=[29.736, 25.168, 25.166, 25.165, 25.164, 25.157, 25.166, 25.305, 25.557, 25.828], "t rola tras"=[30.753, 25.334, 25.325, 25.327, 25.319, 25.312, 25.347, 25.726, 26.292, 26.842], "t amb"=[24.495, 24.289, 24.29, 24.29, 24.295, 24.298, 24.295, 24.293, 24.294, 24.294], "duty cycle"=[24.495, 24.289, 24.29, 24.29, 24.295, 24.298, 24.295, 24.293, 24.294, 24.294]} ("temperature array cluster 2"), "t"=w329, "t1 bobina"=w328, "t2 bobina"=w327, "t freio"=w326, "t rola tras"=w321, "t rola frente"=w320, "t amb"=w313, "duty cycle"=w312) -> (→"temperature array cluster":T2)
        n578 = Bundle By Name(cluster=T9 {"t"=array[506 elements], "torque"=array[506 elements], "ref"=array[506 elements], "lim sup"=array[506 elements], "lim inf"=array[506 elements], "var contr"=array[506 elements]} ("torque array cluster"), "t"=w439, "torque"=w438, "ref"=w437, "lim sup"=w436, "lim inf"=w435, "var contr"=w376) -> (→"torque array cluster":T9)
        n579 = local read "stop geral"() -> (w450:bool)
      }
      n580 = local read "ME"() -> (w72:enum16{"Stand-by", "Ensaiando", "Saindo"})
      n581 = while {
        shift-right: [w912] -> _
        shift-left: w72 -> [w913]
        stop <- w910 stop-if-true
        # "Máquina de estados"
        n582 = case shown="\"Ensaiando\"" w913 {
          tunnel: [w916 w931 enum16{"Stand-by", "Ensaiando", "Saindo"}."Saindo" ("ME")] -> w912
          tunnel: [FALSE ("stop geral") FALSE ("stop geral") TRUE ("stop geral")] -> w911
          frame "Stand-by", Default {
            n583 = flat-sequence {
              tunnel: [w922] -> w916
              frame #0 {
                n584 = while {
                  stop <- w919 stop-if-true
                  n585 = local read "Ensaiando?"() -> (w921:bool)
                  n586 = local read "stop geral"() -> (w920:bool)
                  n587 = Wait (ms)(milliseconds to wait=u32 300) -> ()  [unwired: 1 out]
                  n588 = Or(x=w921, y=w920) -> (x .or. y?=w919:bool)
                }
                n589 = local write "Status de execução"("Rodando" ("Status de execução")) -> ()
              }
              frame #1 {
                n590 = local read "stop geral"() -> (w923:bool)
                n591 = case shown="False" w923 {
                  tunnel: [enum16{"Stand-by", "Ensaiando", "Saindo"}."Ensaiando" ("ME") enum16{"Stand-by", "Ensaiando", "Saindo"}."Saindo" ("ME")] -> w922
                  frame False {
                    n592 = disable-structure shown="Disabled" {
                      frame Disabled {
                        n593 = property on="Tab Control" class="TabCtl (strict)"() -> ("Pages"=w928:refnum<vi>[])  [unwired: 2 in, 2 out]
                        n594 = Index Array(array=w928, index=1) -> (element=w926:refnum<vi>)
                        n595 = property class="Page"(reference=w926, "PageEnb"=T24."Page Disabled & Grayed" ("Page Enabled State")) -> ()  [unwired: 1 in, 2 out]
                      }
                      frame Enabled {
                      }
                    }
                  }
                  frame True {
                  }
                }
              }
            }
          }
          frame "Ensaiando" {
            n596 = flat-sequence {
              tunnel: [enum16{"Stand-by", "Ensaiando", "Saindo"}."Stand-by" ("ME")] -> w931
              frame #0 {
                n597 = local read "Lista de ensaios"() -> (w934:T13)
                n598 = case shown="\"Eficiência (um ponto)\", Default" w934 {
                  frame "Eficiência (um ponto)", Default {
                    n599 = stacked-sequence {
                      frame #0 {
                        # "Inicia o controle da velocidade angular, e espera um tempo"
                        n600 = flat-sequence {
                          frame #0 {
                            n601 = local read "Velocidade angular (RPM)"() -> (w970:dbl)
                            n602 = local write "Referência entrada (RPM)"(w970) -> ()
                          }
                          frame #1 {
                            n603 = property on="Habilitar (RPM)" class="Bool (strict)"("Val(Sgnl)"=TRUE ("Value (Signaling)")) -> ()  [unwired: 2 in, 2 out]
                          }
                          frame #2 {
                            n604 = Wait (ms)(milliseconds to wait=u32 5000) -> ()  [unwired: 1 out]
                          }
                        }
                      }
                      frame #1 {
                        # "Inicia o controle da torque, e espera até que ambas as variáveis estejam em regime permanente"
                        n605 = flat-sequence {
                          tunnel: [w976] -> w973
                          tunnel: w973 -> [w978]
                          frame #0 {
                            n606 = property on="Habilitar (Torque)" class="Bool (strict)"("Val(Sgnl)"=TRUE ("Value (Signaling)")) -> ()  [unwired: 2 in, 2 out]
                            n607 = Wait (ms)(milliseconds to wait=u32 200) -> ()  [unwired: 1 out]
                          }
                          frame #1 {
                            n608 = local read "Torque (mN.m)"() -> (w977:dbl)
                            n609 = local write "Referência entrada (mN.m)"(w977) -> ()
                            n610 = Equal To 0?(x=w977) -> (x = 0?=w976:bool)
                          }
                          frame #2 {
                            n611 = while {
                              tunnel: w978 -> [w979]
                              stop <- w981 stop-if-true
                              n612 = local read "rpm em rp?"() -> (w984:bool)
                              n613 = local read "torque em rp?"() -> (w980:bool)
                              n614 = local read "stop geral"() -> (w982:bool)
                              n615 = Wait (ms)(milliseconds to wait=u32 100) -> ()  [unwired: 1 out]
                              n616 = case shown="False" w979 {
                                tunnel: w984 -> [w986 w989]
                                tunnel: [w986 w988] -> w983
                                tunnel: w980 -> [_ w987]
                                frame True {
                                }
                                frame False {
                                n617 = And(x=w989, y=w987) -> (x .and. y?=w988:bool)
                                }
                              }
                              n618 = Or(x=w983, y=w982) -> (x .or. y?=w981:bool)
                            }
                          }
                          frame #3 {
                            n619 = local read "stop geral"() -> (w990:bool)
                            n620 = case shown="False" w990 {
                              frame False {
                                n621 = Wait (ms)(milliseconds to wait=u32 10000) -> ()  [unwired: 1 out]
                              }
                              frame True {
                              }
                            }
                          }
                        }
                      }
                      frame #2 {
                        # "Realiza as medições de torque, velocidade angular e variáveis elétricas"
                        n622 = flat-sequence {
                          tunnel: [w999] -> w993
                          tunnel: [w1000] -> w995
                          tunnel: w995 -> [w1012]
                          tunnel: [w1011] -> w994
                          tunnel: w993 -> [w1013]
                          tunnel: [w1013] -> w992
                          tunnel: w994 -> [w1015]
                          tunnel: w992 -> [w1016]
                          frame #0 {
                            n623 = local write "Medição contínua? WT230"(TRUE ("Medição contínua?")) -> ()
                            n624 = property on="Realiza medição WT230" class="Bool (strict)"("Val(Sgnl)"=TRUE ("Value (Signaling)")) -> ()  [unwired: 2 in, 2 out]
                          }
                          frame #1 {
                            n625 = call <vilib>:"High Resolution Relative Seconds.vi"() -> ("relative seconds"=w999:dbl)
                            n626 = while {
                              tunnel: w999 -> [w1006]
                              tunnel: [w1001] -> w1000
                              stop <- w1002 stop-if-true
                              n627 = call <vilib>:"High Resolution Relative Seconds.vi"() -> ("relative seconds"=w1007:dbl)
                              n628 = Subtract(x=w1007, y=w1006) -> (x-y=w1005:dbl)
                              n629 = local read "stop geral"() -> (w1004:bool)
                              n630 = Greater?(x=w1005, y="T aquisição") -> (0:w1003:bool)
                              n631 = Wait (ms)(milliseconds to wait=u32 100) -> ()  [unwired: 1 out]
                              n632 = Or(x=w1004, y=w1003) -> (x .or. y?=w1002:bool)
                              n633 = local write "stop aquisition?"(w1003) -> ()
                              n634 = call <vilib>:"High Resolution Relative Seconds.vi"() -> ("relative seconds"=w1001:dbl)
                            }
                          }
                          frame #2 {
                            n635 = Subtract(x=w1012, y=0.5) -> (x-y=w1011:dbl)
                          }
                          frame #3 {
                            n636 = local read "temperature array cluster"() -> (w1014:T2)
                            n637 = local read "torque array cluster"() -> (w1021:T9)
                            n638 = local read "rpm array cluster"() -> (w1022:T6)
                            n639 = local read "watt array cluster"() -> (w1020:T5)
                            n640 = call "rpm_decluster_by_time.vi"("t_final"=w1015, "t_init"=w1016, "rpm array cluster"=w1022) -> ("Dados"=w1031:dbl[][], "Tempo"=w1032:dbl[])  [unwired: 7 in]
                            n641 = call "torque_decluster_by_time.vi"("t_init"=w1016, "torque array cluster"=w1021) -> ("Dados"=w1029:dbl[][], "Tempo"=w1030:dbl[])  [unwired: 8 in]
                            n642 = call "watt_decluster_by_time.vi"("t_init"=w1016, "watt array cluster"=w1020) -> ("Dados"=w1027:dbl[][], "Tempo"=w1028:dbl[])  [unwired: 8 in]
                            n643 = call "temperature_decluster_by_time.vi"("t_init"=w1016, "temperature array cluster"=w1014) -> ("Dados"=w1017:dbl[][], "Tempo"=w1018:dbl[])  [unwired: 8 in]
                            n644 = Build Array (concatenate)(w1032, w1031, w1030, w1029, w1028, w1027, w1018, w1017) -> (w1026:dbl[][])
                            n645 = Transpose 2D Array(2D array=w1026) -> (transposed array=w1025:dbl[][])
                            n646 = Build Path(base path=path "C:/Users/zomer/Desktop/zomer/LabVIEW/dyna_liae/ensaios" ("file path (dialog if empty)"), name or relative path="name or relative path") -> (appended path=w1023:path)
                            n647 = call-poly <vilib>:"Write Delimited Spreadsheet.vi"("file path (dialog if empty)"=w1023, "format (%.3f)"="%.6f", "2D data"=w1025) -> ()  [unwired: 11 in, 2 out]
                          }
                        }
                        n648 = local write "Status de execução"("Eficiência no ponto" ("Status de execução")) -> ()
                      }
                      frame #3 {
                        # "Desativa as malhas de controle"
                        n649 = case shown="False" "manter na condição após ensaio?" {
                          frame False {
                            w1036 = FALSE ("Value (Signaling)")
                            n650 = property on="Habilitar (Torque)" class="Bool (strict)"("Val(Sgnl)"=w1036) -> ()  [unwired: 2 in, 2 out]
                            n651 = property on="Habilitar (RPM)" class="Bool (strict)"("Val(Sgnl)"=w1036) -> ()  [unwired: 2 in, 2 out]
                          }
                          frame True {
                          }
                        }
                        n652 = local write "Medição contínua? WT230"(FALSE ("Medição contínua?")) -> ()
                      }
                    }
                  }
                  frame "Eficiência (um ponto) v2" {
                    n653 = stacked-sequence {
                      frame #0 {
                        # "Inicia o controle da velocidade angular, e espera um tempo"
                        n654 = flat-sequence {
                          frame #0 {
                            n655 = local read "Velocidade angular (RPM)"() -> (w1037:dbl)
                            n656 = local write "Referência entrada (RPM)"(w1037) -> ()
                          }
                          frame #1 {
                            n657 = property on="Habilitar (RPM)" class="Bool (strict)"("Val(Sgnl)"=TRUE ("Value (Signaling)")) -> ()  [unwired: 2 in, 2 out]
                          }
                          frame #2 {
                            n658 = while {
                              stop <- w1039 stop-if-true
                              n659 = local read "rpm em rp?"() -> (w1041:bool)
                              n660 = local read "stop geral"() -> (w1040:bool)
                              n661 = Wait (ms)(milliseconds to wait=u32 100) -> ()  [unwired: 1 out]
                              n662 = Or(x=w1041, y=w1040) -> (x .or. y?=w1039:bool)
                            }
                          }
                          frame #3 {
                            n663 = Wait (ms)(milliseconds to wait=u32 3000) -> ()  [unwired: 1 out]
                          }
                          frame #4 {
                            n664 = call <vilib>:"High Resolution Relative Seconds.vi"() -> ("relative seconds"=w1045:dbl)
                            n665 = while {
                              tunnel: w1045 -> [w1048]
                              tunnel: [w1047] -> w1044 mode=indexing
                              stop <- w1050 stop-if-true
                              n666 = call <vilib>:"High Resolution Relative Seconds.vi"() -> ("relative seconds"=w1054:dbl)
                              n667 = Subtract(x=w1054, y=w1048) -> (x-y=w1053:dbl)
                              n668 = local read "torque mean"() -> (w1047:dbl)
                              n669 = local read "stop geral"() -> (w1052:bool)
                              n670 = Greater?(x=w1053, y=5.0) -> (0:w1051:bool)
                              n671 = Wait (ms)(milliseconds to wait=u32 100) -> ()  [unwired: 1 out]
                              n672 = Or(x=w1052, y=w1051) -> (x .or. y?=w1050:bool)
                            }
                            n673 = call-poly <vilib>:"Mean.vi"("X"=w1044) -> ("mean"=w1046:dbl)  [unwired: 1 out]
                            n674 = local write "Torque à vazio"(w1046) -> ()
                          }
                        }
                      }
                      frame #1 {
                        # "Inicia o controle da torque, e espera até que ambas as variáveis estejam em regime permanente"
                        n675 = flat-sequence {
                          tunnel: [w1060] -> w1056
                          tunnel: w1056 -> [w1061]
                          frame #0 {
                            n676 = property on="Habilitar (Torque)" class="Bool (strict)"("Val(Sgnl)"=TRUE ("Value (Signaling)")) -> ()  [unwired: 2 in, 2 out]
                            n677 = Wait (ms)(milliseconds to wait=u32 200) -> ()  [unwired: 1 out]
                          }
                          frame #1 {
                            n678 = local read "Torque (mN.m)"() -> (w1059:dbl)
                            n679 = Equal To 0?(x=w1059) -> (x = 0?=w1060:bool)
                            n680 = local write "Referência entrada (mN.m)"(w1059) -> ()
                          }
                          frame #2 {
                            n681 = while {
                              tunnel: w1061 -> [w1062]
                              stop <- w1064 stop-if-true
                              n682 = local read "rpm em rp?"() -> (w1067:bool)
                              n683 = local read "torque em rp?"() -> (w1063:bool)
                              n684 = local read "stop geral"() -> (w1065:bool)
                              n685 = Wait (ms)(milliseconds to wait=u32 100) -> ()  [unwired: 1 out]
                              n686 = case shown="False" w1062 {
                                tunnel: w1067 -> [w1069 w1072]
                                tunnel: [w1069 w1071] -> w1066
                                tunnel: w1063 -> [_ w1070]
                                frame True {
                                }
                                frame False {
                                n687 = And(x=w1072, y=w1070) -> (x .and. y?=w1071:bool)
                                }
                              }
                              n688 = Or(x=w1066, y=w1065) -> (x .or. y?=w1064:bool)
                            }
                          }
                          frame #3 {
                            n689 = local read "stop geral"() -> (w1073:bool)
                            n690 = case shown="False" w1073 {
                              frame False {
                                n691 = Wait (ms)(milliseconds to wait=u32 5000) -> ()  [unwired: 1 out]
                              }
                              frame True {
                              }
                            }
                          }
                        }
                      }
                      frame #2 {
                        # "Realiza as medições de torque, velocidade angular e variáveis elétricas"
                        n692 = flat-sequence {
                          tunnel: [w1082] -> w1076
                          tunnel: [w1083] -> w1078
                          tunnel: w1078 -> [w1095]
                          tunnel: [w1094] -> w1077
                          tunnel: w1076 -> [w1096]
                          tunnel: [w1096] -> w1075
                          tunnel: w1077 -> [w1099]
                          tunnel: w1075 -> [w1100]
                          frame #0 {
                            n693 = local write "Medição contínua? WT230"(TRUE ("Medição contínua?")) -> ()
                            n694 = property on="Realiza medição WT230" class="Bool (strict)"("Val(Sgnl)"=TRUE ("Value (Signaling)")) -> ()  [unwired: 2 in, 2 out]
                          }
                          frame #1 {
                            n695 = call <vilib>:"High Resolution Relative Seconds.vi"() -> ("relative seconds"=w1082:dbl)
                            n696 = while {
                              tunnel: w1082 -> [w1090]
                              tunnel: [w1085] -> w1083
                              stop <- w1086 stop-if-true
                              n697 = local read "T aquisição"() -> (w1084:dbl)
                              n698 = call <vilib>:"High Resolution Relative Seconds.vi"() -> ("relative seconds"=w1091:dbl)
                              n699 = Subtract(x=w1091, y=w1090) -> (x-y=w1089:dbl)
                              n700 = local read "stop geral"() -> (w1088:bool)
                              n701 = Greater?(x=w1089, y=w1084) -> (0:w1087:bool)
                              n702 = Wait (ms)(milliseconds to wait=u32 100) -> ()  [unwired: 1 out]
                              n703 = Or(x=w1088, y=w1087) -> (x .or. y?=w1086:bool)
                              n704 = local write "stop aquisition?"(w1087) -> ()
                              n705 = call <vilib>:"High Resolution Relative Seconds.vi"() -> ("relative seconds"=w1085:dbl)
                            }
                          }
                          frame #2 {
                            n706 = Subtract(x=w1095, y=0.5) -> (x-y=w1094:dbl)
                          }
                          frame #3 {
                            n707 = local read "name or relative path"() -> (w1098:string)
                            n708 = local read "temperature array cluster"() -> (w1097:T2)
                            n709 = local read "torque array cluster"() -> (w1104:T9)
                            n710 = local read "rpm array cluster"() -> (w1105:T6)
                            n711 = local read "watt array cluster"() -> (w1103:T5)
                            n712 = call "rpm_decluster_by_time.vi"("t_final"=w1099, "t_init"=w1100, "rpm array cluster"=w1105) -> ("Dados"=w1114:dbl[][], "Tempo"=w1115:dbl[])  [unwired: 7 in]
                            n713 = call "torque_decluster_by_time.vi"("t_init"=w1100, "torque array cluster"=w1104) -> ("Dados"=w1112:dbl[][], "Tempo"=w1113:dbl[])  [unwired: 8 in]
                            n714 = call "watt_decluster_by_time.vi"("t_init"=w1100, "watt array cluster"=w1103) -> ("Dados"=w1110:dbl[][], "Tempo"=w1111:dbl[])  [unwired: 8 in]
                            n715 = call "temperature_decluster_by_time.vi"("t_init"=w1100, "temperature array cluster"=w1097) -> ("Dados"=w1101:dbl[][], "Tempo"=w1102:dbl[])  [unwired: 8 in]
                            n716 = Build Array (concatenate)(w1115, w1114, w1113, w1112, w1111, w1110, w1102, w1101) -> (w1109:dbl[][])
                            n717 = Transpose 2D Array(2D array=w1109) -> (transposed array=w1108:dbl[][])
                            n718 = Build Path(base path=path "C:/Users/zomer/Desktop/zomer/LabVIEW/dyna_liae/ensaios" ("file path (dialog if empty)"), name or relative path=w1098) -> (appended path=w1106:path)
                            n719 = call-poly <vilib>:"Write Delimited Spreadsheet.vi"("file path (dialog if empty)"=w1106, "format (%.3f)"="%.6f", "2D data"=w1108) -> ()  [unwired: 11 in, 2 out]
                          }
                        }
                        n720 = local write "Status de execução"("Eficiência no ponto" ("Status de execução")) -> ()
                      }
                      frame #3 {
                        # "Desativa as malhas de controle"
                        n721 = local read "manter na condição após ensaio?"() -> (w1118:bool)
                        n722 = local write "Torque à vazio"(0.0 ("Torque à vazio")) -> ()
                        n723 = case shown="False" w1118 {
                          frame False {
                            w1120 = FALSE ("Value (Signaling)")
                            n724 = property on="Habilitar (RPM)" class="Bool (strict)"("Val(Sgnl)"=w1120) -> ()  [unwired: 2 in, 2 out]
                            n725 = property on="Habilitar (Torque)" class="Bool (strict)"("Val(Sgnl)"=w1120) -> ()  [unwired: 2 in, 2 out]
                          }
                          frame True {
                            n726 = property on="Habilitar (Torque)" class="Bool (strict)"("Val(Sgnl)"=FALSE ("Value (Signaling)")) -> ()  [unwired: 2 in, 2 out]
                          }
                        }
                        n727 = local write "Medição contínua? WT230"(FALSE ("Medição contínua?")) -> ()
                      }
                    }
                  }
                  frame "Eficiência (múltiplos pontos)" {
                    n728 = stacked-sequence {
                      frame #0 {
                        # "Inicia o controle da velocidade angular e torque, e espera um tempo"
                        n729 = flat-sequence {
                          frame #0 {
                            n730 = local read "Velocidade angular (RPM)"() -> (w1122:dbl)
                            n731 = local write "Referência entrada (RPM)"(w1122) -> ()
                          }
                          frame #1 {
                            n732 = property on="Habilitar (RPM)" class="Bool (strict)"("Val(Sgnl)"=TRUE ("Value (Signaling)")) -> ()  [unwired: 2 in, 2 out]
                          }
                          frame #2 {
                            n733 = Wait (ms)(milliseconds to wait=u32 5000) -> ()  [unwired: 1 out]
                          }
                          frame #3 {
                            n734 = property on="Habilitar (Torque)" class="Bool (strict)"("Val(Sgnl)"=TRUE ("Value (Signaling)")) -> ()  [unwired: 2 in, 2 out]
                            n735 = Wait (ms)(milliseconds to wait=u32 1000) -> ()  [unwired: 1 out]
                          }
                        }
                      }
                      frame #1 {
                        (unwired) u16[] [1, 0, 2, 3] items=["Standard", "Complete", "Symmetric", "Anti Symmetric"]
                        # "Execute a lógica do ensaio"
                        n736 = for {
                          tunnel: "Array modos" -> [w1128] mode=indexing
                          n737 = for {
                            tunnel: "Array frequências" -> [w1130] mode=indexing
                            tunnel: w1128 -> [w1131]
                            n738 = stacked-sequence {
                              tunnel: w1131 -> [w1133 _ _ _ _ _]
                              tunnel: w1130 -> [w1132 _ _ _ _ _]
                              frame #0 {
                                # "Seta os parâmetros do inversor automaticamente para realização dos ensaios em diferentes configurações"
                                n739 = flat-sequence {
                                tunnel: w1133 -> [w1134]
                                tunnel: w1132 -> [w1138]
                                frame #0 {
                                n740 = local read "Parâmetros serial"() -> (w1135:T22)
                                n741 = call "Serial_control.vi"("Enviar número"=w1134, "Função"=T28."Set PWM Mode", "comm cluster"=w1135) -> ()  [unwired: 2 in, 4 out]
                                }
                                frame #1 {
                                n742 = Wait (ms)(milliseconds to wait=u32 1000) -> ()  [unwired: 1 out]
                                }
                                frame #2 {
                                n743 = local read "Parâmetros serial"() -> (w1140:T22)
                                n744 = call "Serial_control.vi"("Enviar número"=w1138, "Função"=T28."Set PWM Frequency", "comm cluster"=w1140) -> ()  [unwired: 2 in, 4 out]
                                }
                                frame #3 {
                                n745 = Wait (ms)(milliseconds to wait=u32 1000) -> ()  [unwired: 1 out]
                                }
                                }
                              }
                              frame #1 {
                                # "Espera até que as variáveis tenham atingido regime permanente"
                                n746 = flat-sequence {
                                tunnel: [w1143] -> w1142
                                tunnel: w1142 -> [w1146]
                                frame #0 {
                                n747 = local read "Torque (mN.m)"() -> (w1144:dbl)
                                n748 = local write "Referência entrada (mN.m)"(w1144) -> ()
                                n749 = Equal To 0?(x=w1144) -> (x = 0?=w1143:bool)
                                }
                                frame #1 {
                                n750 = call <vilib>:"High Resolution Relative Seconds.vi"() -> ("relative seconds"=w1145:dbl)
                                n751 = while {
                                tunnel: w1146 -> [w1155]
                                tunnel: w1145 -> [w1153]
                                stop <- w1149 stop-if-true
                                n752 = local read "rpm em rp?"() -> (w1157:bool)
                                n753 = local read "torque em rp?"() -> (w1156:bool)
                                n754 = local read "stop geral"() -> (w1150:bool)
                                n755 = call <vilib>:"High Resolution Relative Seconds.vi"() -> ("relative seconds"=w1154:dbl)
                                n756 = Wait (ms)(milliseconds to wait=u32 100) -> ()  [unwired: 1 out]
                                n757 = Subtract(x=w1154, y=w1153) -> (x-y=w1152:dbl)
                                n758 = case shown="False" w1155 {
                                tunnel: w1157 -> [w1159 w1162]
                                tunnel: [w1159 w1161] -> w1151
                                tunnel: w1156 -> [_ w1160]
                                frame True {
                                }
                                frame False {
                                n759 = And(x=w1162, y=w1160) -> (x .and. y?=w1161:bool)
                                }
                                }
                                n760 = Greater?(x=w1152, y=30.0) -> (0:w1148:bool)
                                n761 = Compound Arithmetic op=OR(w1151, w1150, w1148) -> (w1149:bool)
                                }
                                }
                                frame #2 {
                                n762 = local read "stop geral"() -> (w1163:bool)
                                n763 = case shown="False" w1163 {
                                frame False {
                                n764 = Wait (ms)(milliseconds to wait=u32 10000) -> ()  [unwired: 1 out]
                                }
                                frame True {
                                }
                                }
                                }
                                }
                              }
                              frame #2 {
                                # "Inicia medição de potência e espera N segundos para finalizar"
                                n765 = flat-sequence {
                                frame #0 {
                                n766 = local write "Medição contínua? WT230"(TRUE ("Medição contínua?")) -> ()
                                n767 = property on="Realiza medição WT230" class="Bool (strict)"("Val(Sgnl)"=TRUE ("Value (Signaling)")) -> ()  [unwired: 2 in, 2 out]
                                }
                                frame #1 {
                                n768 = call <vilib>:"High Resolution Relative Seconds.vi"() -> ("relative seconds"=w1169:dbl)
                                "T init ensaio" <- w1169
                                n769 = while {
                                tunnel: w1169 -> [w1176]
                                tunnel: [w1171] -> w1168
                                stop <- w1172 stop-if-true
                                n770 = local read "T aquisição"() -> (w1170:dbl)
                                n771 = call <vilib>:"High Resolution Relative Seconds.vi"() -> ("relative seconds"=w1177:dbl)
                                n772 = Subtract(x=w1177, y=w1176) -> (x-y=w1175:dbl)
                                n773 = local read "stop geral"() -> (w1174:bool)
                                n774 = Greater?(x=w1175, y=w1170) -> (0:w1173:bool)
                                n775 = Wait (ms)(milliseconds to wait=u32 100) -> ()  [unwired: 1 out]
                                n776 = Or(x=w1174, y=w1173) -> (x .or. y?=w1172:bool)
                                n777 = call <vilib>:"High Resolution Relative Seconds.vi"() -> ("relative seconds"=w1171:dbl)
                                }
                                "T end ensaio" <- w1168
                                }
                                }
                                n778 = local write "Status de execução"("Eficiência no ponto" ("Status de execução")) -> ()
                              }
                              frame #3 {
                                n779 = flat-sequence {
                                tunnel: [w1183] -> w1182
                                tunnel: w1182 -> [w1187]
                                tunnel: [w1187] -> w1181
                                tunnel: w1181 -> [w1190]
                                tunnel: [w1190] -> w1180
                                tunnel: [w1189] -> w1179
                                tunnel: w1180 -> [w1208]
                                tunnel: w1179 -> [w1204]
                                frame #0 {
                                n780 = local read "Parâmetros serial"() -> (w1186:T22)
                                n781 = call "Serial_control.vi"("Message"=T29."Read PWM mode", "Função"=T28."Send Static Message", "comm cluster"=w1186) -> ("translated message"=w1183:string)  [unwired: 2 in, 3 out]
                                }
                                frame #1 {
                                n782 = Wait (ms)(milliseconds to wait=u32 500) -> ()  [unwired: 1 out]
                                }
                                frame #2 {
                                n783 = local read "Parâmetros serial"() -> (w1192:T22)
                                n784 = call "Serial_control.vi"("Message"=T29."Read PWM frequency", "Função"=T28."Send Static Message", "comm cluster"=w1192) -> ("translated message"=w1189:string)  [unwired: 2 in, 3 out]
                                }
                                frame #3 {
                                w1202 = "_" ("string")
                                n785 = local read "Referência entrada (mN.m)"() -> (w1196:dbl)
                                n786 = local read "Referência entrada (RPM)"() -> (w1197:dbl)
                                n787 = local read "name or relative path"() -> (w1195:string)
                                n788 = Search and Replace String(replace all?=TRUE ("replace all? (F)"), input string=w1208, search string=" ", replace string="_" ("replace string (\"\")")) -> (result string=w1212:string)  [unwired: 4 in, 3 out]
                                n789 = Search and Replace String(input string=w1204, search string=" ", replace string="_" ("replace string (\"\")")) -> (result string=w1203:string)  [unwired: 5 in, 3 out]
                                n790 = Number To Decimal String(number=w1196) -> (decimal integer string=w1201:string)  [unwired: 1 in]
                                n791 = Number To Decimal String(number=w1197) -> (decimal integer string=w1200:string)  [unwired: 1 in]
                                n792 = Concatenate Strings(w1212, w1202, w1203, w1202, w1201, "_mNm_" ("string"), w1200, "_RPM_" ("string"), w1195, "_rep" ("string")) -> (→"save name":string)
                                }
                                }
                              }
                              frame #4 {
                                # "Salva os dados"
                                n793 = local read "T init ensaio"() -> (w1221:dbl)
                                n794 = local read "T end ensaio"() -> (w1220:dbl)
                                n795 = Subtract(x=w1220, y=0.5) -> ()  [unwired: 1 out]
                                n796 = local read "temperature array cluster"() -> (w1216:T2)
                                n797 = local read "save name"() -> (w1214:string)
                                n798 = local read "torque array cluster"() -> (w1225:T9)
                                n799 = local read "rpm array cluster"() -> (w1226:T6)
                                n800 = local read "watt array cluster"() -> (w1224:T5)
                                n801 = call "rpm_decluster_by_time.vi"("t_init"=w1221, "rpm array cluster"=w1226) -> ("Dados"=w1234:dbl[][], "Tempo"=w1235:dbl[])  [unwired: 8 in]
                                n802 = call "torque_decluster_by_time.vi"("t_init"=w1221, "torque array cluster"=w1225) -> ("Dados"=w1232:dbl[][], "Tempo"=w1233:dbl[])  [unwired: 8 in]
                                n803 = call "watt_decluster_by_time.vi"("t_init"=w1221, "watt array cluster"=w1224) -> ("Dados"=w1230:dbl[][], "Tempo"=w1231:dbl[])  [unwired: 8 in]
                                n804 = call "temperature_decluster_by_time.vi"("t_init"=w1221, "temperature array cluster"=w1216) -> ("Dados"=w1222:dbl[][], "Tempo"=w1223:dbl[])  [unwired: 8 in]
                                n805 = Concatenate Strings(w1214, ".txt" ("string")) -> (w1215:string)
                                n806 = Build Array (concatenate)(w1235, w1234, w1233, w1232, w1231, w1230, w1223, w1222) -> (w1229:dbl[][])
                                n807 = Transpose 2D Array(2D array=w1229) -> (transposed array=w1228:dbl[][])
                                n808 = Build Path(base path=path "C:/Users/zomer/Desktop/zomer/LabVIEW/dyna_liae/ensaios/aaa" ("file path (dialog if empty)"), name or relative path=w1215) -> (appended path=w1227:path)
                                n809 = call-poly <vilib>:"Write Delimited Spreadsheet.vi"("file path (dialog if empty)"=w1227, "format (%.3f)"="%.6f", "2D data"=w1228) -> ()  [unwired: 11 in, 2 out]
                              }
                              frame #5 {
                                n810 = flat-sequence {
                                frame #0 {
                                n811 = local write "Realiza medição PZ4000"(TRUE ("Realiza medição PZ4000")) -> ()
                                }
                                frame #1 {
                                n812 = local read "save name"() -> (w1238:string)
                                n813 = while {
                                stop <- w1240 continue-if-true
                                n814 = local read "Realiza medição PZ4000"() -> (w1240:bool)
                                n815 = Wait (ms)(milliseconds to wait=u32 100) -> ()  [unwired: 1 out]
                                }
                                n816 = Concatenate Strings(w1238, "_WAV.txt" ("string")) -> (w1239:string)
                                n817 = local write "waveform file name"(w1239) -> ()
                                }
                                frame #2 {
                                n818 = Wait (ms)(milliseconds to wait=u32 5000) -> ()  [unwired: 1 out]
                                }
                                frame #3 {
                                n819 = property on="Salvar waveform" class="Bool (strict)"("Val(Sgnl)"=TRUE ("Value (Signaling)")) -> ()  [unwired: 2 in, 2 out]
                                }
                                }
                              }
                            }
                          }
                        }
                      }
                      frame #2 {
                        n820 = local read "manter na condição após ensaio?"() -> (w1246:bool)
                        n821 = local write "Medição contínua? WT230"(FALSE ("Medição contínua?")) -> ()
                        n822 = case shown="False" w1246 {
                          frame False {
                            w1247 = FALSE ("Value (Signaling)")
                            n823 = property on="Habilitar (Torque)" class="Bool (strict)"("Val(Sgnl)"=w1247) -> ()  [unwired: 2 in, 2 out]
                            n824 = property on="Habilitar (RPM)" class="Bool (strict)"("Val(Sgnl)"=w1247) -> ()  [unwired: 2 in, 2 out]
                          }
                          frame True {
                          }
                        }
                        n825 = local write "stop aquisition?"(TRUE ("stop aquisition?")) -> ()
                      }
                    }
                  }
                }
                n826 = call <vilib>:"High Resolution Relative Seconds.vi"() -> ("relative seconds"=w933:dbl)
                n827 = local write "t0 ensaio"(w933) -> ()
                n828 = local write "Status de execução"("Ensaiando" ("Status de execução")) -> ()
                n829 = local write "stop aquisition?"(FALSE ("stop aquisition?")) -> ()
                n830 = while {
                  stop <- w960 stop-if-true
                  n831 = local read "Lista de ensaios"() -> (w936:T13)
                  n832 = local read "stop aquisition?"() -> (w962:bool)
                  n833 = local read "stop geral"() -> (w961:bool)
                  n834 = Or(x=w961, y=w962) -> (x .or. y?=w960:bool)
                  n835 = case shown="\"Eficiência (um ponto) v2\"" w936 {
                    frame "Eficiência (um ponto)", Default {
                    }
                    frame "Eficiência (um ponto) v2" {
                    }
                  }
                  n836 = local read "watt array cluster"() -> (w952:T5)
                  n837 = local read "rpm array cluster"() -> (w941:T6)
                  n838 = local read "t0 ensaio"() -> (w953:dbl)
                  n839 = call "rpm_decluster_by_time.vi"("t_init"=w953, "rpm array cluster"=w941) -> ("Dados"=w957:dbl[][], "Tempo"=w958:dbl[])  [unwired: 8 in]
                  n840 = Unbundle By Name(w952) -> ("t"=w951:dbl[], "PC(T)"=w946:dbl[])
                  n841 = for {
                    N: 4 -> [_]
                    tunnel: w957 -> [w965] mode=indexing
                    tunnel: w958 -> [w966]
                    tunnel: [w964] -> w959 mode=indexing
                    n842 = Bundle("Tempo"=w966, "Dados"=w965) -> (w964:cluster{"Tempo":dbl[], "Dados":dbl[]})  [unwired: 1 in]
                  }
                  "RPM XY" <- w959
                  n843 = local read "t0 ensaio"() -> (w950:dbl)
                  n844 = local read "torque array cluster"() -> (w940:T9)
                  n845 = Wait (ms)(milliseconds to wait=u32 100) -> ()  [unwired: 1 out]
                  n846 = Subtract(x=w951, y=w950) -> (x-y=w947:dbl[])
                  n847 = local read "t0 ensaio"() -> (w937:dbl)
                  n848 = Greater Than 0?(x=w947) -> (x > 0?=w949:bool[])
                  n849 = Search 1D Array(1D array=w949, element=TRUE) -> (index of element=w948:i32)  [unwired: 1 in]
                  n850 = call "torque_decluster_by_time.vi"("t_init"=w937, "torque array cluster"=w940) -> ("Dados"=w954:dbl[][], "Tempo"=w955:dbl[])  [unwired: 8 in]
                  n851 = Array Subset(array=w947, index=w948) -> (w944:dbl[])  [unwired: 1 in]
                  n852 = Array Subset(array=w946, index=w948) -> (w943:dbl[])  [unwired: 1 in]
                  n853 = for {
                    N: 4 -> [_]
                    tunnel: w954 -> [w968] mode=indexing
                    tunnel: w955 -> [w969]
                    tunnel: [w967] -> w963 mode=indexing
                    n854 = Bundle("Tempo"=w969, "Dados"=w968) -> (w967:cluster{"Tempo":dbl[], "Dados":dbl[]})  [unwired: 1 in]
                  }
                  "Torque XY" <- w963
                  n855 = Bundle(w944, w943) -> (→"Power XY":cluster{dbl[], dbl[]})  [unwired: 1 in]
                }
              }
              frame #1 {
                w1249 = FALSE ("Ensaiando?")
                n856 = disable-structure shown="Disabled" {
                  frame Disabled {
                    n857 = property on="Tab Control" class="TabCtl (strict)"() -> ("Pages"=w1254:refnum<vi>[])  [unwired: 2 in, 2 out]
                    n858 = Index Array(array=w1254, index=1) -> (element=w1253:refnum<vi>)
                    n859 = property class="Page"(reference=w1253, "PageEnb"=T24."Page Enabled" ("Page Enabled State")) -> ()  [unwired: 1 in, 2 out]
                  }
                  frame Enabled {
                  }
                }
                n860 = local write "Ensaiando?"(w1249) -> ()
                n861 = local write "Iniciar ensaio"(w1249) -> ()
                n862 = property on="Iniciar ensaio" class="Bool (strict)"("DisabledEnum"=T23."Enabled" ("Disabled")) -> ()  [unwired: 2 in, 2 out]
              }
            }
          }
          frame "Saindo" {
          }
        }
        n863 = local read "stop geral"() -> (w909:bool)
        n864 = Or(x=w911, y=w909) -> (x .or. y?=w910:bool)
        n865 = Wait (ms)(milliseconds to wait=u32 50) -> ()  [unwired: 1 out]
      }
    }
    frame #3 {
      w1385 = refnum<k21> "resfriamento_freio"  # DAQmx Task Name
      w1386 = FALSE ("stop")
      w1389 = refnum<k21> "alimentacao_inversor"  # DAQmx Task Name
      n866 = disable-structure shown="Enabled" {
        frame Disabled {
          n867 = call <vilib>:"IMAQdx Stop Acquisition.vi"("Session In"=T25 "cam0") -> ("error out"=w1405:errorcluster, "Session Out"=w1407:T25)  [unwired: 9 in]
          n868 = call <vilib>:"IMAQdx Unconfigure Acquisition.vi"("error in"=w1405, "Session In"=w1407) -> ("error out"=w1404:errorcluster, "Session Out"=w1406:T25)  [unwired: 8 out]
          n869 = local read "Image Out"() -> (w1401:T10)
          n870 = call <vilib>:"IMAQdx Close Camera.vi"("error in"=w1404, "Session In"=w1406) -> ("error out"=w1403:errorcluster)  [unwired: 9 in]
          n871 = call "Imaq Dispose"("Image"=w1401, "error in (no error)"=w1403) -> ()  [unwired: 4 in, 1 out]
        }
        frame Enabled {
        }
      }
      n872 = call <instrlib>:"Close.vi"("VISA resource name"=refnum<visa-resource-name> "PZ") -> ()  [unwired: 14 in, 1 out]
      n873 = local write "stop manual"(w1386) -> ()
      n874 = local write "stop geral"(w1386) -> ()
      n875 = local write "stop ensaio"(w1386) -> ()
      n876 = local write "Status de execução"("Finalizado" ("Status de execução")) -> ()
      n877 = property on="Parâmetros serial" class="Clust (strict)"("DisabledEnum"=T23."Enabled" ("Disabled")) -> ()  [unwired: 2 in, 2 out]
      n878 = local read "semaforo medição"() -> (w1379:T11)
      n879 = call <vilib>:"Release Semaphore Reference.vi"("semaphore"=w1379) -> ()  [unwired: 9 in, 2 out]
      n880 = flat-sequence {
        frame #0 {
          n881 = local read "Parâmetros serial"() -> (w1408:T22)
          n882 = call "Serial_control.vi"("Enviar número"=u16 0, "Função"=T26."Set Speed", "comm cluster"=w1408) -> ()  [unwired: 2 in, 4 out]
        }
        frame #1 {
          n883 = local read "Parâmetros serial"() -> (w1412:T22)
          n884 = call "Serial_control.vi"("Função"=T26."End Comm.", "comm cluster"=w1412) -> ()  [unwired: 3 in, 4 out]
        }
      }
      n885 = disable-structure shown="Disabled" {
        frame Disabled {
          w1396 = refnum<k21> "iluminacao"  # DAQmx Task Name
          n886 = call-poly <vilib>:"DAQmx Write.vi"("task/channels in"=w1396, "data"=FALSE) -> ("task out"=w1399:refnum<k21>, "error out"=w1400:errorcluster)  [unwired: 11 in, 1 out]
          n887 = call <vilib>:"DAQmx Stop Task.vi"("task/channels in"=w1399, "error in"=w1400) -> ("task out"=w1398:refnum<k21>, "error out"=w1397:errorcluster)  [unwired: 12 in]
          n888 = call <vilib>:"DAQmx Clear Task.vi"("task in"=w1398, "error in"=w1397) -> ()  [unwired: 13 in, 1 out]
        }
        frame Enabled {
        }
      }
      n889 = call <instrlib>:"Close.vi"("VISA Resource Name"=refnum<visa-resource-name> "Agilent") -> ()  [unwired: 14 in, 1 out]
      n890 = call-poly <vilib>:"DAQmx Write.vi"("task/channels in"=w1385, "data"=FALSE) -> ("task out"=w1382:refnum<k21>, "error out"=w1381:errorcluster)  [unwired: 11 in, 1 out]
      n891 = call-poly <vilib>:"DAQmx Write.vi"("task/channels in"=w1389, "data"=FALSE) -> ("task out"=w1393:refnum<k21>, "error out"=w1394:errorcluster)  [unwired: 11 in, 1 out]
      n892 = call <vilib>:"DAQmx Stop Task.vi"("task/channels in"=w1382, "error in"=w1381) -> ("task out"=w1383:refnum<k21>, "error out"=w1384:errorcluster)  [unwired: 12 in]
      n893 = call <vilib>:"DAQmx Stop Task.vi"("task/channels in"=w1393, "error in"=w1394) -> ("task out"=w1392:refnum<k21>, "error out"=w1391:errorcluster)  [unwired: 12 in]
      n894 = call <vilib>:"DAQmx Clear Task.vi"("task in"=w1383, "error in"=w1384) -> ()  [unwired: 13 in, 1 out]
      n895 = call <vilib>:"DAQmx Clear Task.vi"("task in"=w1392, "error in"=w1391) -> ()  [unwired: 13 in, 1 out]
    }
  }
